vi "Tool detail GUI and STAT 2 collector.vi"(1 "Detail W1":u16, 2 "Detail W2":u16, 3 "LEIN contoller STAT2 data dekoder":i32, 11 "error in (no error)":errorcluster) -> ()   [LabVIEW 2011]
uses:
  Analog value.ctl
  Analog Var Disp 0 sif.ctl
  Status indicator Black Small.ctl
  Digital value.ctl
  Measurments Handling/Digital GUI/Digital Display cluster.ctl
  Measurments Handling/Digital GUI/Digital Disp small indicator.ctl
  Status indicator white.ctl
  Controls/Tristate/Tristate Valve state.ctl
  LEINmaster/Defenitions/LEIN STAT 15 Id system cluster v2.ctl
  LEINmaster/Defenitions/LEIN STAT 14 Debug system cluster.ctl
  LEINmaster/Defenitions/Error_system_def.ctl
  LEINmaster/Defenitions/LEIN stat 1 Stat defenition.ctl
  Tool/List of nodes in tool.ctl
  Tool/Stroker/STroker Raw value indicator.ctl
  LEINmaster/Nodes/Controller local stat2.ctl
  LEINmaster/Nodes/pressure stat2.ctl
  LEINmaster/Nodes/solonoid stat2.ctl
  LEINmaster/Nodes/PSU stat2.ctl
  LEINmaster/Nodes/tensionsub stat2.ctl
  LEINmaster/Status any node.ctl
  LEINmaster/Defenitions/stat2/system status/Stat2 system error.ctl
  LEINmaster/Defenitions/stat2/system status/Stat2 system task info.ctl
  Tool/Tab with tool type tabs.ctl
  LEINmaster/Defenitions/LEIN STAT 15 Id system cluster v2 wo lables.ctl
  <vilib>/Utility/miscctls.llb/LVStringsAndValuesArrayTypeDef.ctl
  emi cndiates/E&S/reate/S&E Event source.ctl
  Events/User Event List.ctl
  LEINmaster/Defenitions/LEIN Structure variations.ctl
  Solenoid Status Override.ctl
  LEINmaster/Defenitions/LEIN stat 14 module array.ctl
  Tool/Variable List Tool Digital.ctl
  Measurments Handling/Common/Variable List Common Analog.ctl
  Measurments Handling/Common/Variable List Common Digital.ctl
  Measurments Handling/Action Analog Handler.ctl
  emi Lib/System 01/0 - General/App/Loop control 2/Private/_emi_SMLoop Control Single.vi
  emi Lib/System 01/0 - General/emi_Read System ID.vi
  emi Lib/System 01/0 - General/App/Loop control 2/Private/_emi_ SMLoop start condition.vi
  emi Lib/System 01/0 - General/App/Loop control 2/Private/_emi_ SMLoop Error Check.vi
  emi Lib/System 01/0 - General/App/Loop control 2/Private/_emi_SMLoop Register new.vi
  emi Lib/System 01/0 - General/S&E reporting/emi_Send S&E Error message.vi
  emi Lib/Basic/0 - General/Error/emi_ Is Error state.vi
  emi Lib/System 01/0 - General/App/Loop control/Private/_emi_GFV Loop Running.vi
  emi Lib/System 01/0 - General/App/Loop control 2/Private/_emi_ SMLoop Restart Counter.vi
  emi Lib/System 01/0 - General/App/Loop control/Private/_emi_GFV stop a loop so it can reset.vi
  emi Lib/System 01/0 - General/App/Loop control 2/Private/_emi_ SMLoop Restart.vi
  emi Lib/System 01/0 - General/App/Loop control/Private/_emi_GFV Loop Linking.vi
  emi Lib/System 01/0 - General/App/Loop control/Private/_emi_GFV Loop Enable.vi
  emi Lib/System 01/0 - General/App/Private/_emi_GFV App Close.vi
  emi Lib/System 01/0 - General/Private/_emi_GFV System ID.vi
  emi Lib/System 01/0 - General/S&E reporting/Private/_emi_S&E Q Generator.vi
  <vilib>/Utility/VariantDataType/GetNumericInfo.vi
panel:
  in  "Close":bool
  out "Tool type:":string
  in  "Tab Control":T1(tab)
  out "Type tab 2":T2
  in  "Send stroker current pos new":bool caption="Solonoid 3 off"
  in  "Stroke pos (mm)":dbl format="%.1f"
  out "Anchor":T3 caption="Solonoid State Anchor"
  out "Solenoid State Stroker":T3 caption="Stroker direction"
  out "Solenoid State Master":T3 caption="Stroker enable"
  in  "Solonoid 1 On":bool
  in  "Solenoid 2 On":bool
  in  "Solenoid 3 On":bool
  in  "Solenoid 1 Off":bool
  in  "Solenoid 2 Off":bool
  in  "Solonoid 3 off":bool
  in  "Send stroker current pos":bool caption="Solonoid 3 off"
  in  "Stroke position to use(mm)":dbl format="%.1f"
  in  "Force ID update":bool caption="Solonoid 3 off"
  out "Main controller":T4 {"LEIN impl. code" format="%02x"; "Serial number" format="%04.0f"; "HW ID" format="%02x"; "FW ID" format="%02x"; "HW REV" format="%02x"; "FW REV" format="%02x"}
  out "Sub nodes":T5[](array[typedef]) {"LEIN implementation code" format="%.0x"; "Serial number" format="%04.0f"; "HW REV" format="%02x"}
  out "Node status array":T6[](array[typedef])
  out "Tool Raw values":T9 {"PSU"."sys register" format="%04x"; "Tension Sub 2"."sys register" format="%04x"; "Tension Sub 1"."sys register" format="%04x"; "Solenoid"."valve status" format="%02x"; "Solenoid"."sys register" format="%04x"; "pressure 2"."sys register" format="%04x"; "pressure 1"."sys register" format="%04x"; "Controller"."High G monitoring" format="%02x"; "Controller"."NA" format="%02x"; "Controller"."GPIO values" format="%02x"; "Controller"."Relay status" format="%02x"; "Controller"."sys register" format="%04x"}
  in  "Clear error":bool
  in  "Node":T15 items=["Stroker Main Controller", "Pressure node 1", "Pressure node 2", "Solenoid node", "PSU", "Tension Sub1", "Tension Sub2"]
  out "Debug received":bool
  out "Error received":bool
  out "Task received":bool
  out "Common Task status":T16
  out "Common error":T17 {"Module error mask" format="%08b"}
  in  "Get Task registers":bool
  in  "Get Error registers":bool
  in  "Get Debug registers":bool
  out "Common Debug data":T18
  out "Additional Task status":string
  out "Additional Error status":string
  out "Additional Debug status":string
  out "System digital values":T19[](array[typedef])
  out "System analog values":T23[](array[typedef]) {"val"."Value" format="%#.1f"}
  # "Direct solenoid control"
  # "Solenoid status override"
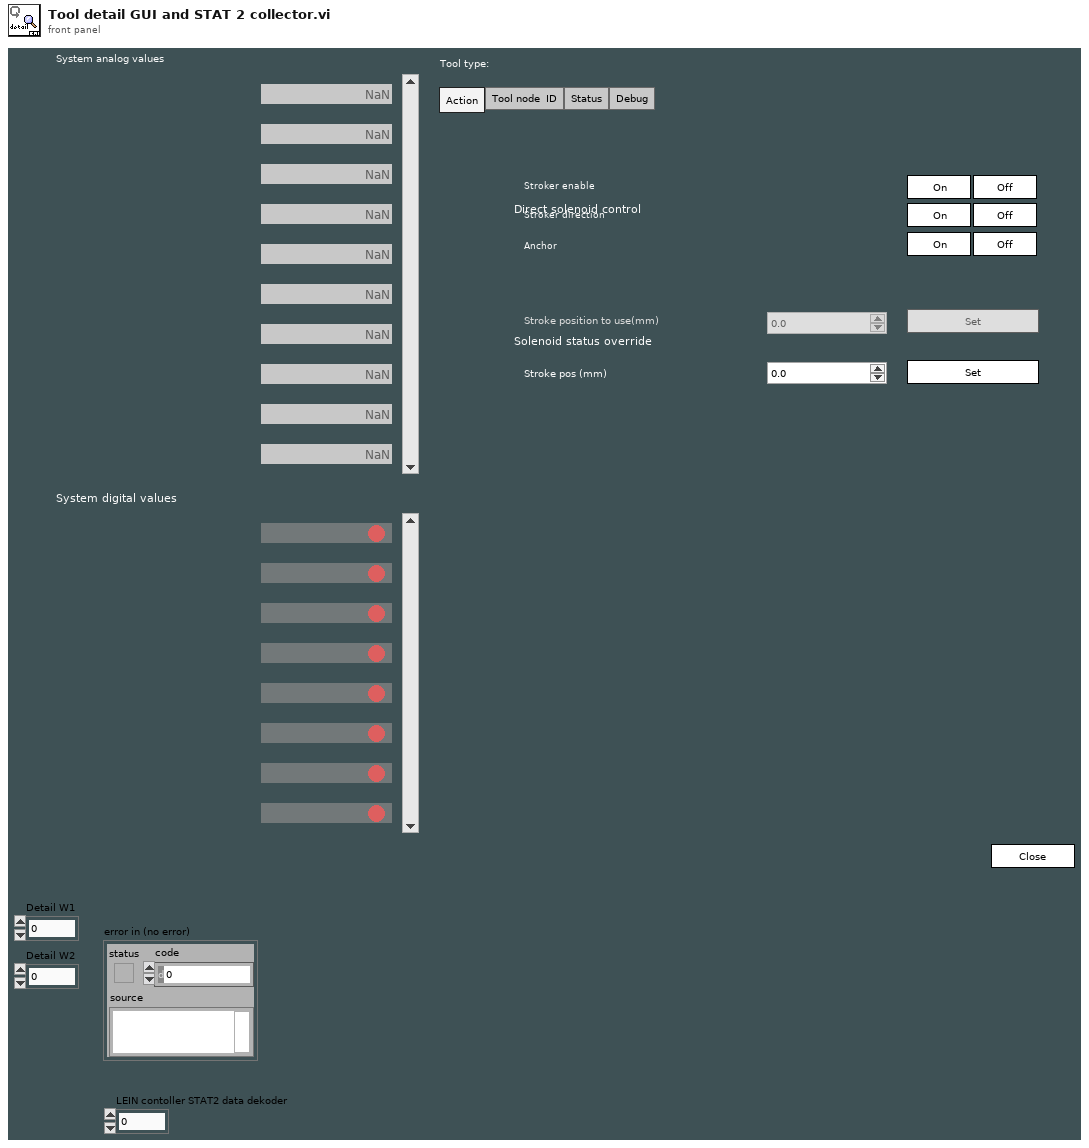
[diagram p1: front panel]
types:
  T1 = enum32{"Action", "Tool node  ID", "Status", "Debug"}
  T2 = typedef "Tab with tool type tabs.ctl" = enum32{"Stroker", "Driller", "Tractor"}
  T3 = typedef "Tristate Valve state.ctl" = u16
  T4 = typedef "LEIN STAT 15 Id system cluster v2.ctl" = cluster{"LEIN version":u8, "LEIN impl. code":u8, "Serial number":u16, "Project":u16, "HW ID":u8, "FW ID":u8, "HW REV":u8, "FW REV":u8}
  T5 = typedef "LEIN STAT 15 Id system cluster v2 wo lables.ctl" = cluster{"LEIN version":u8, "LEIN implementation code":u8, "Serial number":u16, "Project":u16, "HW ID":u8, "FW ID":u8, "HW REV":u8, "FW REV":u8}
  T6 = typedef "Status any node.ctl" = cluster{"Name":string, "Connected":bool, "Stopped":bool, "Error":T7, "Task":T8}
  T7 = typedef "Stat2 system error.ctl" = cluster{"Error":bool, "Has had error":bool, "Com. issue":bool}
  T8 = typedef "Stat2 system task info.ctl" = cluster{"Task":bool, "Task error":bool, "Task cnt.":u8, "Job 0":bool, "User":bool}
  T9 = typedef "STroker Raw value indicator.ctl" = cluster{"Controller":T10, "pressure 1":T11, "pressure 2":T11, "Solenoid":T12, "PSU":T13, "Tension Sub 1":T14, "Tension Sub 2":T14, "Pos override used":bool}
  T10 = typedef "Controller local stat2.ctl" = cluster{"sys register":u16, "temperature":u16, "Input voltage":u16, "Input Current":u16, "Accelerometer ch0":u16, "Accelerometer ch1":u16, "Accelerometer ch2":u16, "Relay status":u8, "GPIO values":u8, "Sensor 1":i32, "Sensor 2":i32, "NA":u8, "High G monitoring":u8}
  T11 = typedef "pressure stat2.ctl" = cluster{"sys register":u16, "temperature":u16, "Pressure":u16, "osctun":u8}
  T12 = typedef "solonoid stat2.ctl" = cluster{"sys register":u16, "temperature":u16, "Position":i16, "monitor state":u8, "valve status":u8}
  T13 = typedef "PSU stat2.ctl" = cluster{"sys register":u16, "temperature":u16, "HV Voltage in":u16, "Main Voltage out":u16, "Main Current out":u16}
  T14 = typedef "tensionsub stat2.ctl" = cluster{"sys register":u16, "temperature":u16, "Tension":i16, "osctun":u8}
  T15 = typedef "List of nodes in tool.ctl" = u16
  T16 = typedef "LEIN stat 1 Stat defenition.ctl" = cluster{"Task ID":u8, "Task counter":u8, "Task result code":u8, "reserved":u8}
  T17 = typedef "Error_system_def.ctl" = cluster{"Uptime(minutes)":u16, "Com state 1 (crc/Tx)":u8, "Com state 2 (bit timing /Rx)":u8, "System error code":u8, "Module error mask":u8}
  T18 = typedef "LEIN STAT 14 Debug system cluster.ctl" = cluster{"Max handler call interval":u16, "Messages received":u16, "Valid messages received":u16, "Replies sent":u16, "Nack sent":u16}
  T19 = typedef "Digital value.ctl" = cluster{"Name":string, "Val":T20}
  T20 = typedef "Digital Display cluster.ctl" = cluster{"ON/OFF TEXT":string, "Val":T21, "Status":T22}
  T21 = typedef "Digital Disp small indicator.ctl" = u16
  T22 = typedef "Status indicator white.ctl" = u16
  T23 = typedef "Analog value.ctl" = cluster{"Name":string, "val":T24}
  T24 = typedef "Analog Var Disp 0 sif.ctl" = cluster{"Value":dbl, "Unit":string, "Status":T25}
  T25 = typedef "Status indicator Black Small.ctl" = u16
  T26 = typedef "LVStringsAndValuesArrayTypeDef.ctl" = cluster{"String":string, "Value":ext}[]
  T27 = typedef "Variable List Tool Digital.ctl" = enum16{"Tool Error Controller", "Tool Stopped Controller", "Tool Relay 1", "Tool Relay 2", "Tool Both Relays", "Tool node Pressure 1", "Tool Error Pressure 1", "Tool Stopped Pressure 1", "Tool node Pressure 2", "Tool Error Pressure 2", "Tool Stopped Pressure 2", "Tool node Solenoid", "Tool Error Solenoid", "Tool Stopped Solenoid", "Tool Solenoid 1", "Tool Solenoid 2", "Tool Solenoid 3", "Tool node PSU", "Tool Error PSU", "Tool Stopped PSU", "Upper Tension Sub", "Tool Error Upper Tension Sub", "Tool Stopped Upper Tension Sub", "Lower Tension Sub", "Tool Error Lower Tension Sub", "Tool Stopped Lower Tension Sub", "Stroke Target seeking", "Stroke Moving Out", "Stroke Moving Inn", "Stroke valves set for Out", "Stroke valves set for In", "Stroke In (force)", "Stroke Out (force)", "Stroke Force decreasing(in)", "Stroke Force decreasing(out)", "Stroke Force change not correct", "Stroke SLIPS established P1", "Stroke SLIPS established P2", "Stroke SLIPS established", "Stroke Pressure Monitor Ongoing", "Stroke Pressure Monitor Ending ", "Tool Stroke enable Valve", "Tool Stroke direction Valve", "Tool Anchor Valve", "Stroker Var19 - Reserved", "Stroker Var20 - Reserved", "Stroker Var21 - Reserved", "Stroker Var22 - Reserved", "Stroker Var23 - Reserved", "Stroker Var24 - Reserved", "Tractor Var1 - Reserved", "Tractor Var2 - Reserved", "Tractor Var3 - Reserved", "Tractor Var4 - Reserved", "Tractor Var5 - Reserved", "Tractor Var6 - Reserved", "Tractor Var7 - Reserved", "Tractor Var8 - Reserved", "Oil filling mode", "Mill Bit Direction", "Position control", "Anchor", "Driller Var5 - Reserved", "Driller Var6 - Reserved", "Driller Var7 - Reserved", "Driller Var8 - Reserved"}
  T28 = typedef "S&E Event source.ctl" = enum16{"User", "Instrument", "Application", "Windows"}
  T29 = enum16{"big-endian, network order", "native, host order", "little-endian"}
  T30 = typedef "LEIN custom reply Q.ctl" = refnum<queue>
  T31 = typedef "_emi_ SMLoop sates.ctl" = enum16{"Init", "Standby", "Start", "Normal Operation", "Stop", "Error Handling", "End", "Post"}
  T32 = typedef "Options  All pages and custom.ctl" = cluster{"P 1 (App)":T33, "P 2":T34, "P 3":T35, "P 4":T38, "P 5":T43, "P 6 (Err)":T44, "P 7 (Expert)":T45, "P 8 (Depth)":T47, "C 1":T48, "C 2":T49}
  T33 = typedef "Options Page 1 (App).ctl" = cluster{"Result files":path, "PCP Interface":string, "Tractor/Stroker Interface":string, "Tractor Interface":string, "Modem Status Interface":string, "Audible Alarm":bool, "Force alarm on Technical":bool, "Force alarm on HH":bool, "Force alarm on LL":bool, "Force alarm on H":bool, "Force alarm on L":bool}
  T34 = typedef "Options Page 2.ctl" = cluster{"Solenoid & Relay latching time":u16, "Tractor relay 1":dbl, "Tractor relay 2":dbl, "Tractor Solenoid limit":dbl}
  T35 = typedef "Options Page 3.ctl" = cluster{"Min resistance":dbl, "Max resistance":dbl, "Head voltage range":T36, "Max voltage jump":dbl, "Maximum resistance change":dbl, "Start Telemetry Voltage":dbl, "Start Telemetry Timeout":dbl, "Start Motor Voltage":dbl, "Stop Motor Voltage":dbl, "Pass Mode Warning Voltage":dbl, "Relay Switch Voltage":dbl, "Relay Status Loss Voltage":dbl, "Samples to average":i32, "PSU type DO NOT USE":T37, "Magna OVP":dbl, "Magna Current Limit":dbl}
  T36 = typedef "PCP type List.ctl" = enum16{"0 - 350V", "0 - 450V", "0 - 600V"}
  T37 = typedef "PSU Type.ctl" = enum16{"Unipower", "Magna 8.3A", "Magna 12A", "None"}
  T38 = typedef "Options Page 4.ctl" = cluster{"Solenoid & Relay latching time":u16, "Stroker relay 1":dbl, "Stroker Relay 2":dbl, "Stroker Solenoid limit":dbl, "Force det.":T39, "Stroke force lim.":dbl, "Anchor Enabled Pressure":dbl, "Tacometer puls":dbl, "Default anchor behavior":T40, "Default stroker behavior":T41, "Default stroker force limit (tonne)":dbl, "Slips Size":T42}
  T39 = typedef "Stroke force selector.ctl" = enum16{"Stroke in = node 1", "Strok out = node 1"}
  T40 = typedef "Default anchor behavior.ctl" = enum16{"Do nothing", "Set Anchor", "Release Anchor"}
  T41 = typedef "Default stroker behavior.ctl" = enum16{"Do nothing", "Stop", "Go Out", "Go In"}
  T42 = typedef "Slips Type Radio.ctl" = enum32{"No Selection", "338 MRS", "3,9 MRS"}
  T43 = typedef "Options Page 5.ctl" = cluster{"Solenoid & Relay latching time":u16, "Driller relay 1":dbl, "Driller Relay 2":dbl, "Driller  Solenoid limit":dbl}
  T44 = typedef "Options Page 6 (Err).ctl" = cluster{"Error and event files":path}
  T45 = typedef "Options Page 7 (Expert).ctl" = cluster{"Show Debug":bool, "Log debug messages":bool, "Additional debug messages":bool, "Start Beagle with Simulator data":bool, "Workshop mode":bool, "Modem baud":u16, "enumCANCOM":bool, "Modem sim":T46, "Telemetry Timeout Disable":i32, "Buffer size":i32, "Upd regular data":bool, "Cable comp":cluster{"VMOD1 Voltage(V)":dbl, "VMOD2 Voltage(V)":dbl}}
  T46 = typedef "Modem simulation setup.ctl" = cluster{"Modem dealay sim":bool, "Sim baud Tx":u16, "Bit Error fraction Tx":dbl, "Sim baud Rx":u16, "Bit Error fraction Rx":dbl}
  T47 = typedef "Options Page 8 (Depth).ctl" = cluster{"Winch Spool Circumference":dbl, "Winch Pulses per Revolution":dbl, "Current Depth":dbl}
  T48 = typedef "Options Custom 1.ctl" = cluster{"Depth Updated":bool, "Depth Offset":dbl}
  T49 = typedef "Options Custom 2.ctl" = cluster{"Placeholder":bool}
  T50 = typedef "List of tools.ctl" = enum16{"Stroker", "Driller", "Tractor"}
  T51 = typedef "User Event List.ctl" = enum16{"ESCAPE", "HV ON", "HV OFF", "HV SP Start adjusting", "HV SP Adjusted", "Sequence Started", "Stop Tool Operation", "Start Telemetry Operation", "Start Motor Operation", "Stroker Activated", "Driller Activated", "Tractor Activated", "Reset Telemetry", "Stop Telemetry", "Stop Motor Operation", "Cable Resistance Updated", "Cable Resistance Update Failed", "String Check Recording Started", "String Check Recording Stopped", "STROKER tool: Stroke enable Solenoid ON", "STROKER tool: Stroke enable Solenoid OFF", "STROKER tool: Stroke direction Solenoid ON", "STROKER tool: Stroke direction Solenoid OFF", "STROKER tool: Anchor Solenoid ON", "STROKER tool: Anchor Solenoid OFF", "Stroker - Set force and pressure to ZERO", "Stroker - Set tension subs to ZERO", "Mono Relay ON - PASS mode", "Hepta Relay ON - PASS mode", "Mono Relay OFF - MOTOR mode", "Hepta Relay OFF - MOTOR mode", "Relays set to passenger mode", "Relays set to motor mode", "Tractor - Set Tension Subs to ZERO", "High-G monitoring Stop", "High-G data retreival requested", "High-G data stop retreival requested", "High-G data retreived", "STROKER tool: Stroker position override sent", "Stroker Stop", "Stroker Extend", "Stroker Retract", "Stroker go to Position", "Controller Stop command", "Node clear error", "STROKER tool: Stroke stop homing", "STROKER tool: Start Monitoring", "STROKER tool: Stop Monitoring", "Sequence start", "Sequence stop", "Sequence stopped", "Sequence step approved", "Sequence action", "Failed sequence step, Retry", "Failed sequence step, Continue", "Failed sequence step, Abort", "Run Started", "Run Stopped"}
  T52 = typedef "LEIN Structure variations.ctl" = enum16{"LEIN08", "LEIN31", "LEIN63"}
  T53 = typedef "LEIN CMD Cluster.ctl" = cluster{"SID":u8, "ANF":bool, "CMD":T54, "DATA":u8[]}
  T54 = typedef "LEIN CMD List.ctl" = enum8{"ACTI", "TASK", "RES0", "STAT", "RES1", "RES2", "RES3", "USER"}
  T55 = typedef "Solenoid Status Override.ctl" = u8
  T56 = typedef "LEIN stat 14 module array.ctl" = u8[]
  T57 = typedef "Expected STAT lenght cluster.ctl" = cluster{"LEIN 0(error)":u16, "LEIN 1(Task)":u16, "LEIN 2(stat2)":u16, "LEIN 14(Debug)":u16, "LEIN 15(ID)":u16}
  T58 = typedef "Status Digitalish.ctl" = enum16{"NA", "False", "True"}
  T59 = typedef "Fixed Analog Channel Definition.ctl" = cluster{"ID":u16, "Name":string, "Quantity":T60, "Unit":string, "Maximum upd":T61, "Comment":string, "Help file Name":string, "Help file Section ":string, "Category":T62, "User adjustable Scaling":bool, "Default Scaling":T63, "Default Unit":i32, "Classification":T64}
  T60 = typedef "Quantity enum.ctl" = enum16{"NA", "Acceleration", "Angle", "Current", "Force", "Distance", "Pressure", "Resistance", "Rotational Speed", "Speed", "Temperature", "Tension", "Torque", "Voltage", "Weight"}
  T61 = typedef "Update frequensies.ctl" = enum16{"2 Hz", "1 Hz", "0.1 Hz"}
  T62 = typedef "Channel catagory Enum.ctl" = enum16{"No Category", "Power", "Temperature", "Pressure"}
  T63 = typedef "Scaling.ctl" = cluster{"Gain":dbl, "Offset":dbl}
  T64 = typedef "Channel Classification Enum.ctl" = enum16{"Basic", "Advanced", "Expert", "Unused"}
  T65 = typedef "Fixed Digital Channel Definition.ctl" = cluster{"ID":u16, "Name":string, "NA Text":string, "Off Text":string, "On Text":string, "Maximum upd":T61, "Comment":string, "Help file Name":string, "Help file Section ":string, "Catagory":T62, "In use":bool}
  T66 = typedef "Variable List Common Digital.ctl" = enum16{"PCP Connected", "PCP PC Control", "HV PSU connected", "HV PSU HV Active", "Modem Connected", "Tool Connected", "CanBus interface"}
  T67 = typedef "Variable List Common Analog.ctl" = enum16{"HVPSU Head Voltage", "HVPSU TS Voltage", "HVPSU Current", "PCP Cable Resistance", "Winch Depth", "Winch Line Speed", "Winch Wire Tension"}
  T68 = typedef "Action Analog Handler.ctl" = enum16{"GET value", "GET Single Frequenzy", "GET All Values", "GET Waveform", "Get Numb Var", "SET Value", "START Buffer", "REG Variable", "BUF size(total antal sekund)", "PULS", "Get a Value at time", "Set initial waveform"}
  T69 = cluster{"notifier out":refnum<notifier>, "Ana com":i32, "Dig com":i32, "Time of last valid tool data":u32}
  T70 = typedef "STAT2 data carrier type aware.ctl" = cluster{"Tool":T50, "Data":variant}
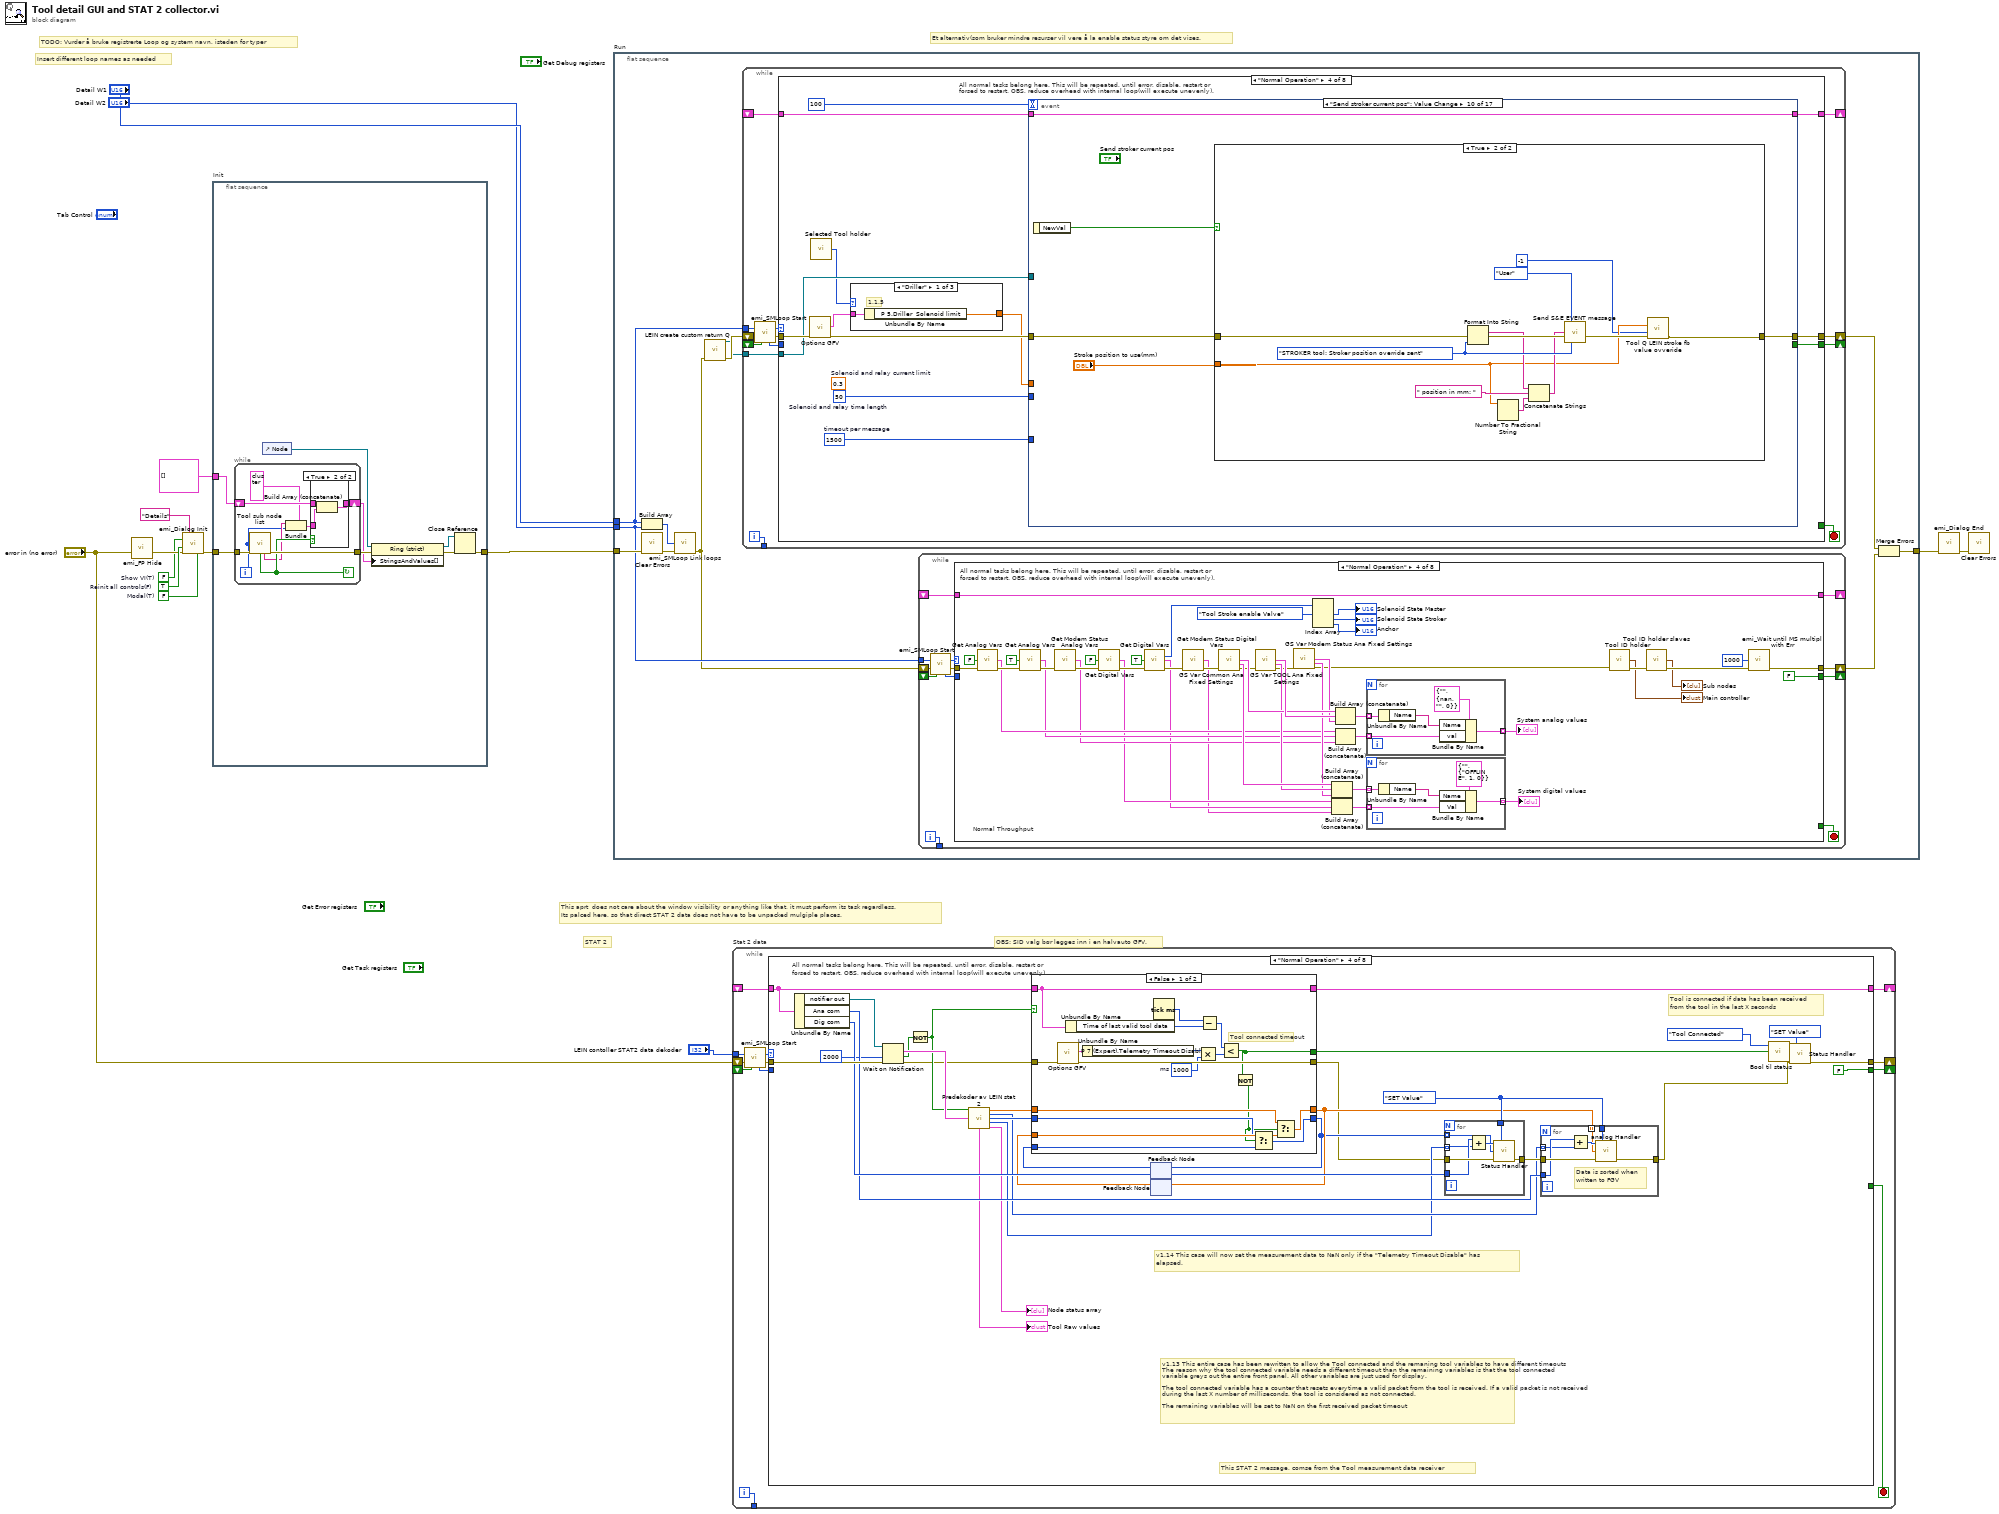
[diagram p0: block diagram]
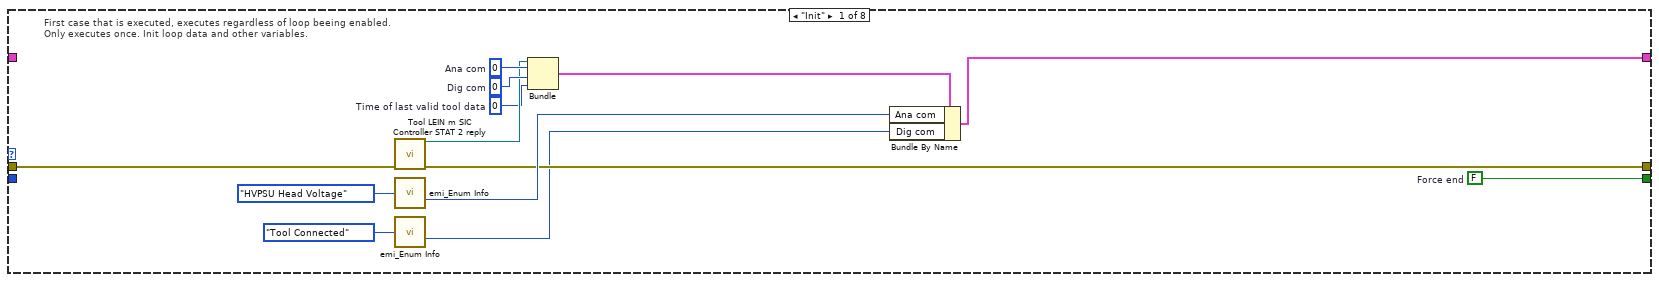
[diagram p2: hidden frame]
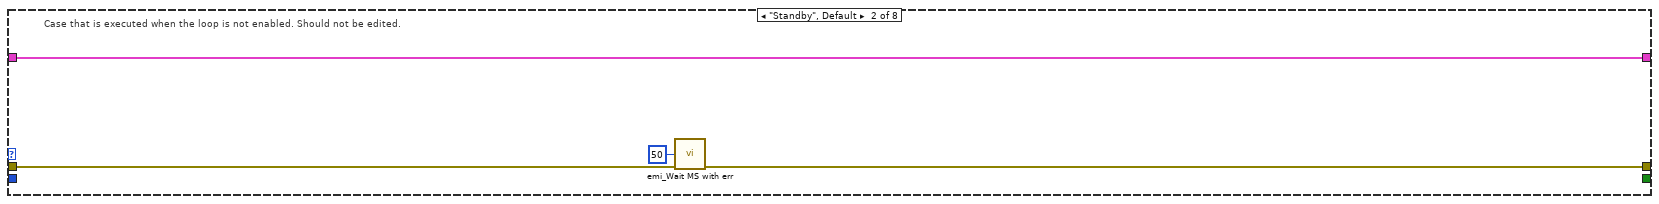
[diagram p3: hidden frame]
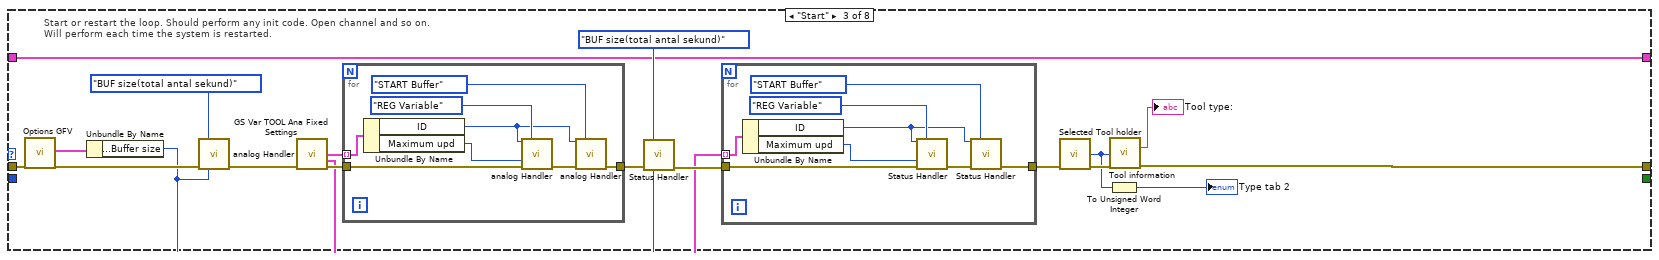
[diagram p4: hidden frame]
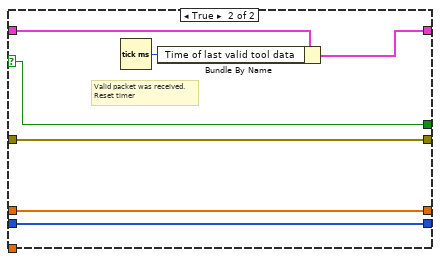
[diagram p5: hidden frame]
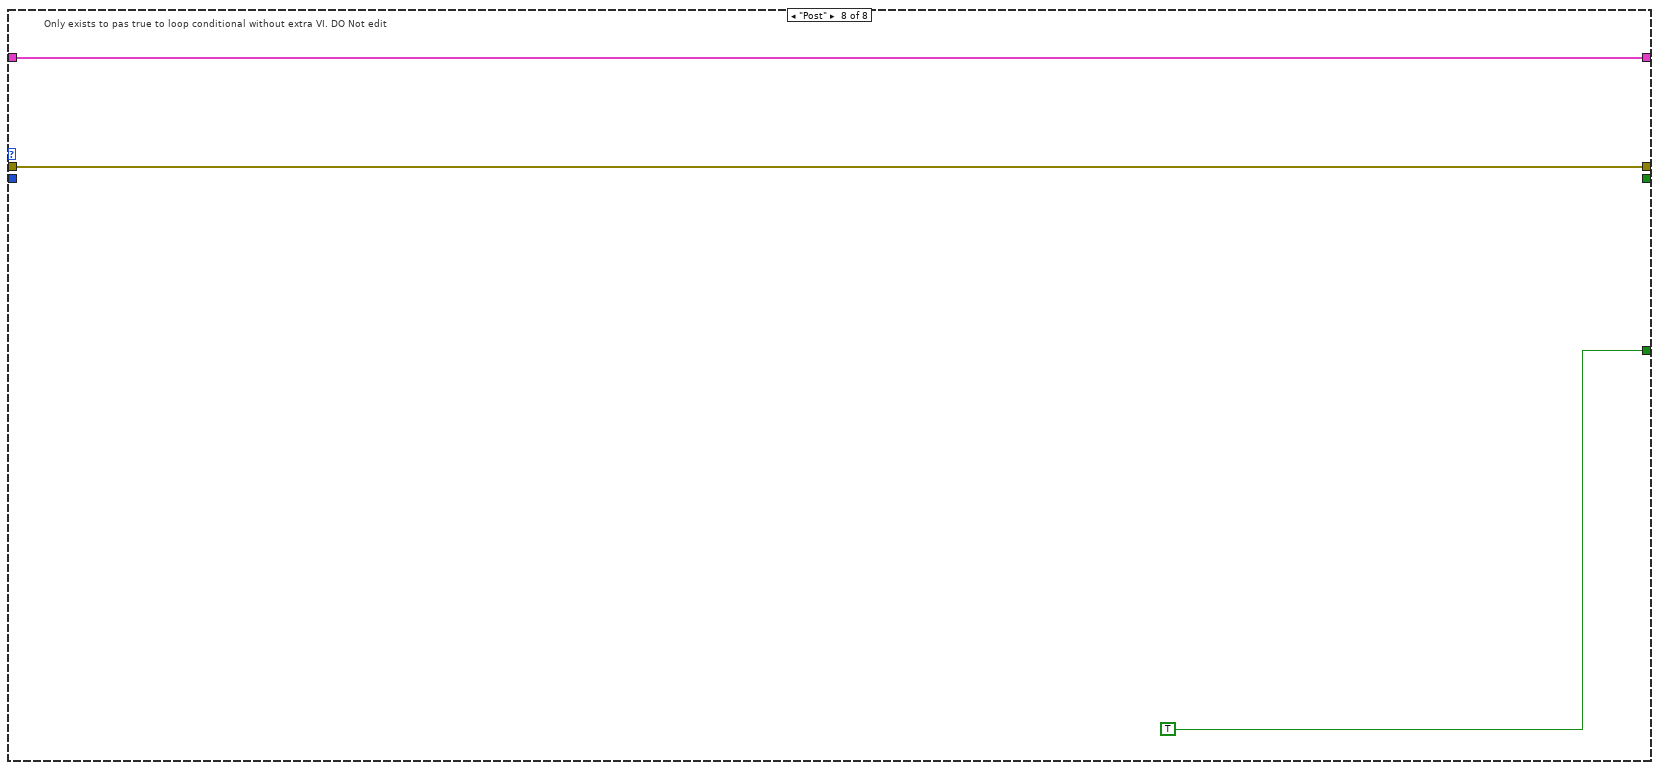
[diagram p9: hidden frame]
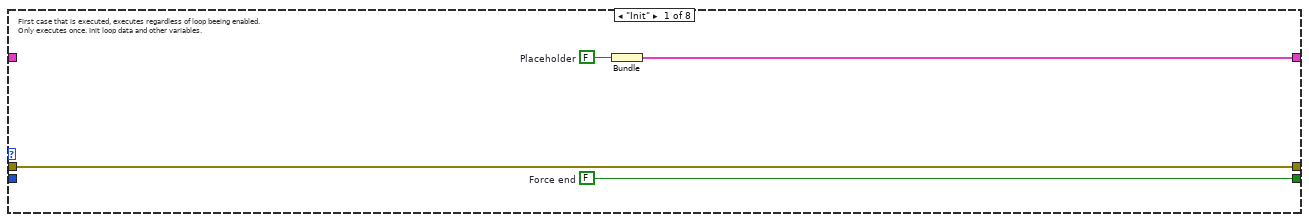
[diagram p11: hidden frame]
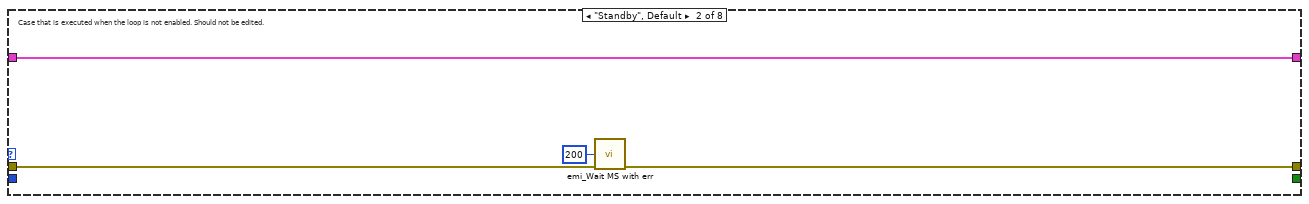
[diagram p12: hidden frame]
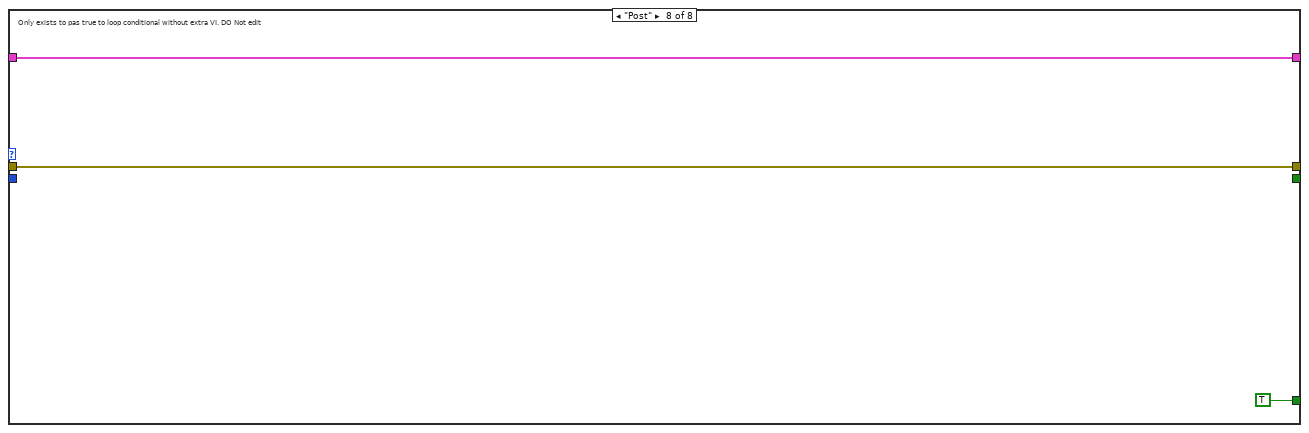
[diagram p17: hidden frame]
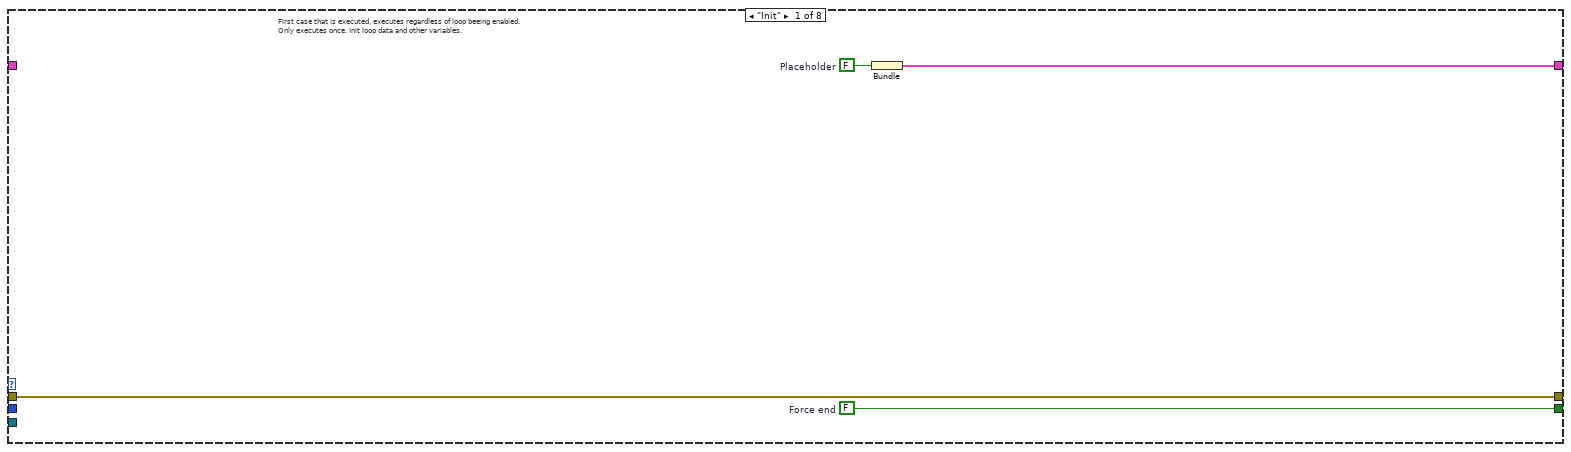
[diagram p18: hidden frame]
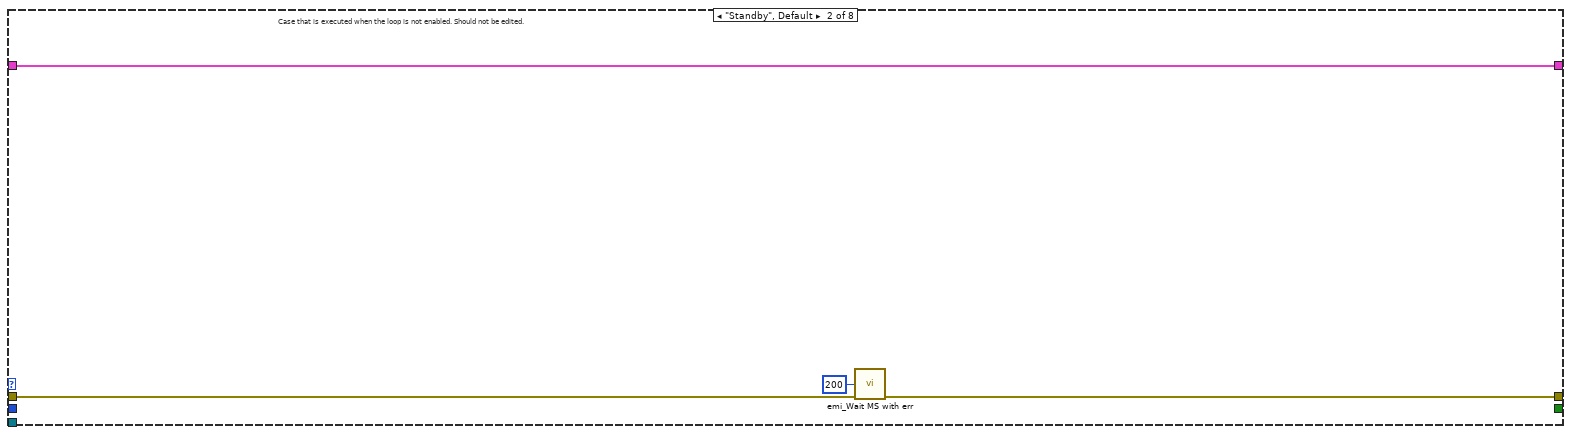
[diagram p19: hidden frame]
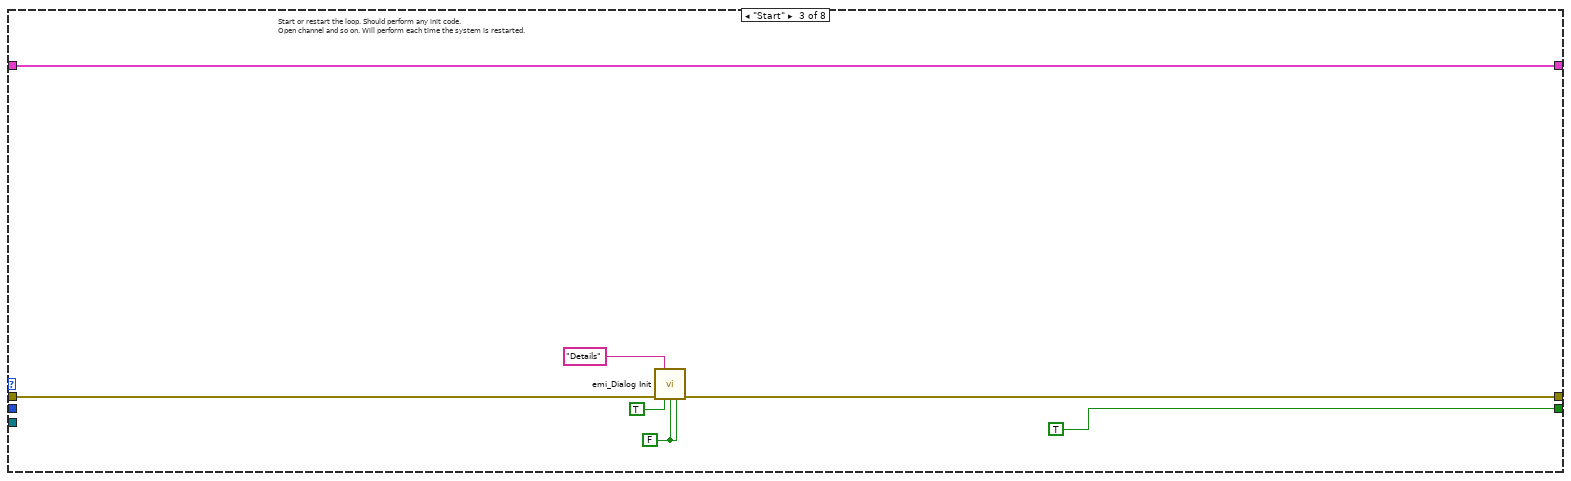
[diagram p20: hidden frame]
diagram:
  w9 = FALSE  # Show VI(T)
  w12 = TRUE  # Reinit all controls(F)
  w13 = FALSE  # Modal(T)
  # "This aprt  does not care about the window visibility or anything like that, it must perform its task regardless.\nIts palced here, so that direct STAT 2 data does not have to be unpacked mulgiple places."
  # "STAT 2"
  # "OBS: SID valg bør legges inn i en halvauto GFV."
  # "Et alternativ(som bruker mindre resurser vil vere å la enable status styre om det vises."
  # "TODO: Vurder å bruke registrerte Loop og system navn, isteden for typer"
  # "Insert different loop names as needed"
  n1 = call "emi_FP Hide.vi"("error in (no error)"="error in (no error)") -> ("error out"=w11:errorcluster)  [unwired: 13 in, 1 out]
  n2 = call "emi_Dialog Init.vi"("Header String(\"\")"="Details" ("Header String(\"\")"), "Show VI(T)"=w9, "Reinit all controls(F)"=w12, "error in"=w11, "Modal(T)"=w13) -> ("error out"=w10:errorcluster)  [unwired: 10 in]
  n3 = flat-sequence "Init" {
    tunnel: [w20] -> w7
    tunnel: w10 -> [w17]
    tunnel: T26 [] ("Strings And Values []") -> [w16]
    frame #0 {
      n4 = while {
        tunnel: [w30] -> w18
        tunnel: w17 -> [w31]
        shift-right: [w28] -> w15
        shift-left: w16 -> [w27]
        i -> [w24]
        stop <- w29 continue-if-true
        n5 = call "Tool sub node list.vi"("Tool node"=w24, "error in (no error)"=w31) -> ("node registered"=w29:bool, "Node name"=w25:string, "error out"=w30:errorcluster)  [unwired: 6 in, 5 out]
        n6 = Bundle(cluster=cluster{"String":string, "Value":ext} {"String"="", "Value"=0.0}, "String"=w25, "Value"=w24) -> (w23:cluster{"String":string, "Value":ext})
        n7 = case shown="True" w29 {
          tunnel: [w32 w34] -> w28
          tunnel: w27 -> [w32 w35]
          tunnel: w23 -> [_ w33]
          frame False {
          }
          frame True {
            n8 = Build Array (concatenate)(w35, w33) -> (w34:T26)
          }
        }
      }
      n9 = control-ref of="Node"() -> (w19:refnum<vi>)
      n10 = property class="Ring (strict)"(reference=w19, error in=w18, "StringsAndValues[]"=w15) -> (reference out=w21:refnum<vi>, error out=w22:errorcluster)
      n11 = Close Reference(reference=w21, error in (no error)=w22) -> (error out=w20:errorcluster)
    }
  }
  n12 = flat-sequence "Run" {
    tunnel: w7 -> [w46]
    tunnel: [w43] -> w8
    tunnel: "Detail W1" -> [w41]
    tunnel: "Detail W2" -> [w40]
    frame #0 {
      n13 = Build Array(w41, w40) -> (w39:u16[])
      n14 = call <vilib>:"Clear Errors.vi"("error in (no error)"=w46) -> ("error out"=w42:errorcluster)  [unwired: 6 in]
      n15 = call "emi_SMLoop Link loops.vi"("Loop IDS"=w39, "error in (no error)"=w42) -> ("error out"=w38:errorcluster)  [unwired: 13 in]
      n16 = call "LEIN create custom return Q.vi"("error in (no error)"=w38) -> ("LEIN custom reply Q"=w36:T30, "error out"=w37:errorcluster)  [unwired: 13 in]
      n17 = while {
        shift-right: [w145] -> _
        shift-left: _ -> [w141]
        shift-right: [w143] -> w45
        shift-left: w37 -> [w139]
        tunnel: [w142] -> _
        shift-right: [w140] -> _
        shift-left: _ -> [w135]
        tunnel: w41 -> [w136]
        tunnel: w36 -> [w133]
        i -> [w142]
        stop <- w144 stop-if-true
        n18 = call "emi_SMLoop Start.vi"("Loop ID"=w136, "error in (no error)"=w139, "Force Stop(F)"=w135) -> ("Loop command"=w137:T31, "error out"=w138:errorcluster, "Loop ID out"=w134:i32)  [unwired: 10 in]
        n19 = case shown="\"Normal Operation\"" w137 {
          tunnel: [w148 w150 w160 w171 w565 w580 w581 w584] -> w145
          tunnel: [_ _ _ _ _ _ _ TRUE] -> w144
          tunnel: w138 -> [w149 w152 w158 w173 w564 w579 w582 w585]
          tunnel: [w149 w151 w159 w172 w560 w579 w582 w585] -> w143
          tunnel: w141 -> [_ w150 w160 w170 w565 w580 w581 w584]
          tunnel: [w146 _ TRUE ("Discard?") w169 _ _ _ _] -> w140
          tunnel: w134 -> [_ _ _ _ w563 _ _ _]
          tunnel: w133 -> [_ _ _ w168 _ _ _ _]
          frame "Init" {
            w146 = FALSE  # Force end
            w147 = FALSE  # Placeholder
            # "First case that is executed, executes regardless of loop beeing enabled.\nOnly executes once. Init loop data and other variables."
            n20 = Bundle("Placeholder"=w147) -> (w148:cluster{"Placeholder":bool})  [unwired: 1 in]
          }
          frame "Standby", Default {
            # "Case that is executed when the loop is not enabled. Should not be edited."
            n21 = call "emi_Wait MS with err.vi"("milliseconds to wait(0)"=u32 200, "error in (no error)"=w152) -> ("error out"=w151:errorcluster)  [unwired: 13 in]
          }
          frame "Start" {
            w155 = FALSE ("Set BG Color(T)")
            # "Start or restart the loop. Should perform any init code. \nOpen channel and so on. Will perform each time the system is restarted."
            n22 = call "emi_Dialog Init.vi"("Header String(\"\")"="Details" ("Header String(\"\")"), "error in"=w158, "Center in bottom FP(T)"=TRUE, "Set BG Color(T)"=w155, "Modal(T)"=w155) -> ("error out"=w159:errorcluster)  [unwired: 10 in]
          }
          frame "Normal Operation" {
            w165 = 1500  # timeout per message
            w166 = u16 50  # Solenoid and relay time length
            (unwired) 0.3  # Solenoid and relay current limit
            # "All normal tasks belong here. This will be repeated, until error, disable, restart or\nforsed to restart. OBS, reduce overhead with internal loop(will execute unevenly)."
            n23 = call "Options GFV.vi"("error in (no error)"=w173) -> ("Options"=w163:T32, "error out"=w164:errorcluster)  [unwired: 16 in, 1 out]
            n24 = call "Selected Tool holder.vi"() -> ("Tool out"=w161:T50)  [unwired: 14 in, 1 out]
            n25 = case shown="\"Driller\"" w161 {
              tunnel: w163 -> [w175 w177 w179]
              tunnel: [w174 w176 w178] -> w162
              frame "Driller" {
                # "1.1.5"
                n26 = Unbundle By Name(w175) -> ("P 5.Driller  Solenoid limit"=w174:dbl)
              }
              frame "Tractor" {
                # "1.1.5"
                n27 = Unbundle By Name(w177) -> ("P 2.Tractor relay 2"=w176:dbl)
              }
              frame "Stroker" {
                # "1.1.5"
                n28 = Unbundle By Name(w179) -> ("P 4.Stroker Solenoid limit"=w178:dbl)
              }
            }
            n29 = event shown="[9] \"Send stroker current pos\": Value Change" {
              selector: _ -> [_ _ _ _ _ _ _ _ _ _ _ _ _ _ _ _ _]
              dyn-events: _ -> [_ _ _ _ _ _ _ _ _ _ _ _ _ _ _ _ _]
              timeout: 100 -> [_ _ _ _ _ _ _ _ _ _ _ _ _ _ _ _ _]
              tunnel: w164 -> [w180 w184 w189 w211 w233 w255 w274 w299 w321 w350 w368 w395 w401 w448 w495 w515 w558]
              tunnel: w170 -> [w182 w185 w191 w213 w235 w257 w279 w301 w323 w352 w370 w396 w403 w450 w497 w517 w559]
              tunnel: [w182 w185 w191 w213 w235 w257 w279 w301 w323 w352 w370 w396 w403 w450 w497 w517 w559] -> w171
              tunnel: [w180 w184 w190 w212 w234 w256 w278 w300 w322 w351 w369 w395 w402 w449 w496 w516 w558] -> w172
              tunnel: [w181 w183 _ _ _ _ _ _ _ _ _ _ _ _ _ _ _] -> w169
              tunnel: w162 -> [_ _ w187 w209 w231 w253 w276 w297 w319 _ _ _ _ _ _ _ _]
              tunnel: w166 -> [_ _ w186 w208 w230 w252 w275 w296 w318 _ _ _ _ _ _ _ _]
              tunnel: w168 -> [_ _ _ _ _ _ _ _ _ _ _ _ w399 w446 w493 w513 _]
              tunnel: w165 -> [_ _ _ _ _ _ _ _ _ _ _ _ w398 w445 w492 w512 _]
              event Panel Close? {
                w181 = TRUE ("Discard?")
                # "Ellers varierer det om \nDebug Synlig/ikke Synlig huskes(\nalt etter om options vises etterpå)"
                n30 = event-data() -> ()  [unwired: 1 in, 3 out]
                n31 = event-data("Discard?"=w181) -> ()  [unwired: 1 in, 1 out]
              }
              event "Close": Value Change {
                n32 = event-data() -> ("NewVal"=w183:bool)  [unwired: 1 in]
              }
              event "Solenoid 1 Off": Value Change {
                n33 = event-data() -> ("NewVal"=w188:bool)  [unwired: 1 in]
                n34 = case shown="False" w188 {
                  tunnel: [w192 w206] -> w190
                  tunnel: w189 -> [w192 w199]
                  tunnel: w187 -> [_ w205]
                  tunnel: w186 -> [_ w204]
                  frame False {
                  }
                  frame True {
                    w197 = T15 3 items=["Main Controller", "Pressure node 1", "Pressure node 2", "Solenoid node"] ("Node")
                    w200 = User_Event_List."STROKER tool: Stroke enable Solenoid OFF" ("User Events")
                    n35 = Format Into String(error in=w199, w200) -> (resulting string=w201:string, error out=w202:errorcluster)  [unwired: 2 in]
                    n36 = call "Send S&E EVENT message.vi"("Event Source(user)"=S&E_Event_source."User", "Event Description"=w201, "error in (no error)"=w202, "Loc Sub ID/Event ID(No ID)"=w200) -> ("error out"=w198:errorcluster)  [unwired: 10 in, 1 out]
                    n37 = call "Selected Tool holder.vi"() -> ("Tool out"=w196:T50, "error out"=w195:errorcluster)  [unwired: 14 in]
                    n38 = call "Tool information.vi"("Tool in"=w196, "error in (no error)"=w195) -> ("Main node address"=w193:u8)  [unwired: 10 in, 3 out]
                    n39 = call "Tool sub node list.vi"("Tool node"=w197) -> ("SID"=w194:u8)  [unwired: 7 in, 7 out]
                    n40 = call "Tool Q LEIN solonoid valve task.vi"("Main Controller ID"=w193, "Solonoid ID"=w194, "current limit(0.2A)"=w205, "outpuyt channel"=u8 1, "time (50 ms)"=w204, "error in (no error)"=w198) -> ("error out"=w206:errorcluster)  [unwired: 8 in, 1 out]
                  }
                }
              }
              event "Solonoid 1 On": Value Change {
                n41 = event-data() -> ("NewVal"=w210:bool)  [unwired: 1 in]
                n42 = case shown="True" w210 {
                  tunnel: [w214 w228] -> w212
                  tunnel: w211 -> [w214 w221]
                  tunnel: w209 -> [_ w227]
                  tunnel: w208 -> [_ w226]
                  frame False {
                  }
                  frame True {
                    w219 = T15 3 items=["Main Controller", "Pressure node 1", "Pressure node 2", "Solenoid node"] ("Node")
                    w222 = User_Event_List."STROKER tool: Stroke enable Solenoid ON" ("User Events")
                    n43 = call "Selected Tool holder.vi"() -> ("Tool out"=w217:T50, "error out"=w216:errorcluster)  [unwired: 14 in]
                    n44 = call "Tool information.vi"("Tool in"=w217, "error in (no error)"=w216) -> ("Main node address"=w215:u8)  [unwired: 10 in, 3 out]
                    n45 = Format Into String(error in=w221, w222) -> (resulting string=w223:string, error out=w224:errorcluster)  [unwired: 2 in]
                    n46 = call "Send S&E EVENT message.vi"("Event Source(user)"=S&E_Event_source."User", "Event Description"=w223, "error in (no error)"=w224, "Loc Sub ID/Event ID(No ID)"=w222) -> ("error out"=w220:errorcluster)  [unwired: 10 in, 1 out]
                    n47 = call "Tool sub node list.vi"("Tool node"=w219) -> ("SID"=w218:u8)  [unwired: 7 in, 7 out]
                    n48 = call "Tool Q LEIN solonoid valve task.vi"("Main Controller ID"=w215, "Solonoid ID"=w218, "current limit(0.2A)"=w227, "outpuyt channel"=u8 0, "time (50 ms)"=w226, "error in (no error)"=w220) -> ("error out"=w228:errorcluster)  [unwired: 8 in, 1 out]
                  }
                }
              }
              event "Solenoid 2 On": Value Change {
                n49 = event-data() -> ("NewVal"=w232:bool)  [unwired: 1 in]
                n50 = case shown="True" w232 {
                  tunnel: [w236 w250] -> w234
                  tunnel: w233 -> [w236 w243]
                  tunnel: w231 -> [_ w249]
                  tunnel: w230 -> [_ w248]
                  frame False {
                  }
                  frame True {
                    w241 = T15 3 items=["Main Controller", "Pressure node 1", "Pressure node 2", "Solenoid node"] ("Node")
                    w244 = User_Event_List."STROKER tool: Stroke direction Solenoid ON" ("User Events")
                    n51 = call "Selected Tool holder.vi"() -> ("Tool out"=w240:T50, "error out"=w239:errorcluster)  [unwired: 14 in]
                    n52 = call "Tool sub node list.vi"("Tool node"=w241) -> ("SID"=w238:u8)  [unwired: 7 in, 7 out]
                    n53 = call "Tool information.vi"("Tool in"=w240, "error in (no error)"=w239) -> ("Main node address"=w237:u8)  [unwired: 10 in, 3 out]
                    n54 = Format Into String(error in=w243, w244) -> (resulting string=w245:string, error out=w246:errorcluster)  [unwired: 2 in]
                    n55 = call "Send S&E EVENT message.vi"("Event Source(user)"=S&E_Event_source."User", "Event Description"=w245, "error in (no error)"=w246, "Loc Sub ID/Event ID(No ID)"=w244) -> ("error out"=w242:errorcluster)  [unwired: 10 in, 1 out]
                    n56 = call "Tool Q LEIN solonoid valve task.vi"("Main Controller ID"=w237, "Solonoid ID"=w238, "current limit(0.2A)"=w249, "outpuyt channel"=u8 2, "time (50 ms)"=w248, "error in (no error)"=w242) -> ("error out"=w250:errorcluster)  [unwired: 8 in, 1 out]
                  }
                }
              }
              event "Solenoid 2 Off": Value Change {
                n57 = event-data() -> ("NewVal"=w254:bool)  [unwired: 1 in]
                n58 = case shown="True" w254 {
                  tunnel: [w258 w272] -> w256
                  tunnel: w255 -> [w258 w265]
                  tunnel: w253 -> [_ w271]
                  tunnel: w252 -> [_ w270]
                  frame False {
                  }
                  frame True {
                    w263 = T15 3 items=["Main Controller", "Pressure node 1", "Pressure node 2", "Solenoid node"] ("Node")
                    w266 = User_Event_List."STROKER tool: Stroke direction Solenoid OFF" ("User Events")
                    n59 = call "Selected Tool holder.vi"() -> ("Tool out"=w262:T50, "error out"=w261:errorcluster)  [unwired: 14 in]
                    n60 = call "Tool sub node list.vi"("Tool node"=w263) -> ("SID"=w260:u8)  [unwired: 7 in, 7 out]
                    n61 = call "Tool information.vi"("Tool in"=w262, "error in (no error)"=w261) -> ("Main node address"=w259:u8)  [unwired: 10 in, 3 out]
                    n62 = Format Into String(error in=w265, w266) -> (resulting string=w267:string, error out=w268:errorcluster)  [unwired: 2 in]
                    n63 = call "Send S&E EVENT message.vi"("Event Source(user)"=S&E_Event_source."User", "Event Description"=w267, "error in (no error)"=w268, "Loc Sub ID/Event ID(No ID)"=w266) -> ("error out"=w264:errorcluster)  [unwired: 10 in, 1 out]
                    n64 = call "Tool Q LEIN solonoid valve task.vi"("Main Controller ID"=w259, "Solonoid ID"=w260, "current limit(0.2A)"=w271, "outpuyt channel"=u8 3, "time (50 ms)"=w270, "error in (no error)"=w264) -> ("error out"=w272:errorcluster)  [unwired: 8 in, 1 out]
                  }
                }
              }
              event "Solenoid 3 On": Value Change {
                n65 = event-data() -> ("NewVal"=w277:bool)  [unwired: 1 in]
                n66 = case shown="True" w277 {
                  tunnel: [w280 w294] -> w278
                  tunnel: w274 -> [w280 w286]
                  tunnel: w276 -> [_ w293]
                  tunnel: w275 -> [_ w292]
                  frame False {
                  }
                  frame True {
                    w285 = T15 3 items=["Main Controller", "Pressure node 1", "Pressure node 2", "Solenoid node"] ("Node")
                    w288 = User_Event_List."STROKER tool: Anchor Solenoid ON" ("User Events")
                    n67 = call "Selected Tool holder.vi"() -> ("Tool out"=w284:T50, "error out"=w283:errorcluster)  [unwired: 14 in]
                    n68 = call "Tool sub node list.vi"("Tool node"=w285) -> ("SID"=w282:u8)  [unwired: 7 in, 7 out]
                    n69 = call "Tool information.vi"("Tool in"=w284, "error in (no error)"=w283) -> ("Main node address"=w281:u8)  [unwired: 10 in, 3 out]
                    n70 = Format Into String(error in=w286, w288) -> (resulting string=w289:string, error out=w290:errorcluster)  [unwired: 2 in]
                    n71 = call "Send S&E EVENT message.vi"("Event Source(user)"=S&E_Event_source."User", "Event Description"=w289, "error in (no error)"=w290, "Loc Sub ID/Event ID(No ID)"=w288) -> ("error out"=w287:errorcluster)  [unwired: 10 in, 1 out]
                    n72 = call "Tool Q LEIN solonoid valve task.vi"("Main Controller ID"=w281, "Solonoid ID"=w282, "current limit(0.2A)"=w293, "outpuyt channel"=u8 4, "time (50 ms)"=w292, "error in (no error)"=w287) -> ("error out"=w294:errorcluster)  [unwired: 8 in, 1 out]
                  }
                }
              }
              event "Solonoid 3 off": Value Change {
                n73 = event-data() -> ("NewVal"=w298:bool)  [unwired: 1 in]
                n74 = case shown="True" w298 {
                  tunnel: [w302 w316] -> w300
                  tunnel: w299 -> [w302 w309]
                  tunnel: w297 -> [_ w315]
                  tunnel: w296 -> [_ w314]
                  frame False {
                  }
                  frame True {
                    w307 = T15 3 items=["Main Controller", "Pressure node 1", "Pressure node 2", "Solenoid node"] ("Node")
                    w310 = User_Event_List."STROKER tool: Anchor Solenoid OFF" ("User Events")
                    n75 = call "Selected Tool holder.vi"() -> ("Tool out"=w306:T50, "error out"=w305:errorcluster)  [unwired: 14 in]
                    n76 = Format Into String(error in=w309, w310) -> (resulting string=w311:string, error out=w312:errorcluster)  [unwired: 2 in]
                    n77 = call "Tool information.vi"("Tool in"=w306, "error in (no error)"=w305) -> ("Main node address"=w303:u8)  [unwired: 10 in, 3 out]
                    n78 = call "Send S&E EVENT message.vi"("Event Source(user)"=S&E_Event_source."User", "Event Description"=w311, "error in (no error)"=w312, "Loc Sub ID/Event ID(No ID)"=w310) -> ("error out"=w308:errorcluster)  [unwired: 10 in, 1 out]
                    n79 = call "Tool sub node list.vi"("Tool node"=w307) -> ("SID"=w304:u8)  [unwired: 7 in, 7 out]
                    n80 = call "Tool Q LEIN solonoid valve task.vi"("Main Controller ID"=w303, "Solonoid ID"=w304, "current limit(0.2A)"=w315, "outpuyt channel"=u8 5, "time (50 ms)"=w314, "error in (no error)"=w308) -> ("error out"=w316:errorcluster)  [unwired: 8 in, 1 out]
                  }
                }
              }
              event "Force ID update": Value Change {
                n81 = event-data() -> ("NewVal"=w320:bool)  [unwired: 1 in]
                n82 = case shown="True" w320 {
                  tunnel: [w324 w332] -> w322
                  tunnel: w321 -> [w324 w331]
                  tunnel: w319 -> [_ _]
                  tunnel: w318 -> [_ _]
                  frame False {
                  }
                  frame True {
                    w338 = u16 60 ("Expected LEN")
                    w337 = LEIN_Structure_variations."LEIN63" ("LEIN Variation")
                    n83 = call "Get node version Q.vi"("error in"=w331) -> ("LEIN custom reply Q"=w330:T30, "error out"=w327:errorcluster)  [unwired: 13 in]
                    n84 = call "Selected Tool holder.vi"("error in (no error)"=w327) -> ("Tool out"=w329:T50, "error out"=w328:errorcluster)  [unwired: 13 in]
                    n85 = call "Tool information.vi"("Tool in"=w329, "error in (no error)"=w328) -> ("Main node address"=w325:u8, "error out"=w326:errorcluster)  [unwired: 10 in, 2 out]
                    n86 = call "LEIN CMD read STATs by len.vi"("SID"=w325, "LEIN Variation"=w337, "Expected LEN"=w338, "STAT ID"=u8 15, "error in"=w326) -> ("STATs"=w335:T53[], "error out"=w340:errorcluster)  [unwired: 9 in]
                    n87 = call "LEIN CMD read STATs by len.vi"("SID"=w325, "LEIN Variation"=w337, "Expected LEN"=w338, "STAT ID"=u8 5, "error in"=w340) -> ("STATs"=w336:T53[], "error out"=w334:errorcluster)  [unwired: 9 in]
                    n88 = Build Array (concatenate)(w335, w336) -> (w333:T53[])
                    n89 = for {
                      tunnel: [w347] -> w332
                      tunnel: w334 -> [w346]
                      tunnel: w333 -> [w345] mode=indexing
                      tunnel: w330 -> [w342]
                      n90 = call "LEIN Q Uniqe command.vi"("LEIN custom reply Q"=w342, "Retry on err (F)"=TRUE, "Custom Q(F)"=TRUE, "CMD"=w345, "error in"=w346) -> ("error out"=w347:errorcluster)  [unwired: 10 in]
                    }
                  }
                }
              }
              event "Send stroker current pos": Value Change {
                n91 = event-data() -> ("NewVal"=w349:bool)  [unwired: 1 in]
                n92 = case shown="True" w349 {
                  tunnel: [w353 w356] -> w351
                  tunnel: w350 -> [w353 w362]
                  tunnel: "Stroke position to use(mm)" -> [_ w355]
                  frame False {
                  }
                  frame True {
                    w363 = User_Event_List."STROKER tool: Stroker position override sent" ("User Events")
                    n93 = Format Into String(error in=w362, w363) -> (resulting string=w361:string, error out=w364:errorcluster)  [unwired: 2 in]
                    n94 = Number To Fractional String(number=w355) -> (F-format string=w358:string)  [unwired: 3 in]
                    n95 = Concatenate Strings(w361, " position in mm: ", w358) -> (w360:string)
                    n96 = call "Send S&E EVENT message.vi"("Event Source(user)"=S&E_Event_source."User", "Event Description"=w360, "error in (no error)"=w364, "Loc Sub ID/Event ID(No ID)"=w363) -> ("error out"=w357:errorcluster)  [unwired: 10 in, 1 out]
                    n97 = call "Tool Q LEIN stroke fb value ovveride.vi"("stroke value(mm)"=w355, "Serial number(any number(-1))"=i16 -1, "error in (no error)"=w357) -> ("error out"=w356:errorcluster)  [unwired: 12 in]
                  }
                }
              }
              event "Send stroker current pos new": Value Change {
                n98 = event-data() -> ("NewVal"=w367:bool)  [unwired: 1 in]
                n99 = case shown="True" w367 {
                  tunnel: [w371 w378] -> w369
                  tunnel: w368 -> [w371 w384]
                  tunnel: "Stroke pos (mm)" -> [_ w377]
                  frame False {
                  }
                  frame True {
                    w373 = T55 3 items=["Don't change"=3, "On"=1, "Off"=2, "Unknown"=0] ("Stroker enable")
                    w374 = T55 3 items=["Don't change"=3, "On"=1, "Off"=2, "Unknown"=0] ("Stroker direction")
                    w375 = T55 3 items=["Don't change"=3, "On"=1, "Off"=2, "Unknown"=0] ("Anchor")
                    w385 = User_Event_List."STROKER tool: Stroker position override sent" ("User Events")
                    n100 = Format Into String(error in=w384, w385) -> (resulting string=w383:string, error out=w386:errorcluster)  [unwired: 2 in]
                    n101 = Number To Fractional String(number=w377) -> (F-format string=w380:string)  [unwired: 3 in]
                    n102 = Concatenate Strings(w383, " position in mm: ", w380) -> (w382:string)
                    n103 = call "Send S&E EVENT message.vi"("Event Source(user)"=S&E_Event_source."User", "Event Description"=w382, "error in (no error)"=w386, "Loc Sub ID/Event ID(No ID)"=w385) -> ("error out"=w379:errorcluster)  [unwired: 10 in, 1 out]
                    n104 = call "Tool Q LEIN stroke fb value ovveride new.vi"("stroke value(mm)"=w377, "Pos Change"=TRUE, "Serial number(any number(-1))"=i16 -1, "error in (no error)"=w379, "Solenoid 3"=w375, "Solenoid 2"=w374, "Solenoid 1"=w373) -> ("error out"=w378:errorcluster)  [unwired: 8 in]
                  }
                }
              }
              event Value Change {
                w388 = ""
                (unwired) T56 [] ("FW module status codes")
                n105 = event-data() -> ()  [unwired: 1 in, 1 out]
                n106 = local write "Additional Task status"(w388) -> ()
                n107 = local write "Additional Error status"(w388) -> ()
                n108 = local write "Additional Debug status"(w388) -> ()
                "Common error" <- T17 {"Uptime(minutes)"=0, "Com state 1 (crc/Tx)"=0, "Com state 2 (bit timing /Rx)"=0, "System error code"=0, "Module error mask"=0} ("Common error")
                "Common Task status" <- T16 {"Task ID"=0, "Task counter"=0, "Task result code"=0, "reserved"=0} ("Common Task status")
                "Task received" <- FALSE ("Task received")
                "Error received" <- FALSE ("Error received")
                "Debug received" <- FALSE ("Debug received")
                "Common Debug data" <- T18 {"Max handler call interval"=0, "Messages received"=0, "Valid messages received"=0, "Replies sent"=0, "Nack sent"=0} ("Common debug data")
              }
              event "Get Task registers": Value Change {
                n109 = event-data() -> ("NewVal"=w400:bool)  [unwired: 1 in]
                n110 = case shown="True" w400 {
                  tunnel: [w404 w436] -> w402
                  tunnel: w401 -> [w404 w437]
                  tunnel: w399 -> [_ w429]
                  tunnel: w398 -> [_ w424]
                  tunnel: "Node" -> [_ w423]
                  frame False {
                  }
                  frame True {
                    w410 = T16 {"Task ID"=0, "Task counter"=0, "Task result code"=0, "reserved"=0} ("Common Task status")
                    n111 = call <vilib>:"Set Busy.vi"("error in (no error)"=w437) -> ("error out"=w432:errorcluster)  [unwired: 9 in, 1 out]
                    n112 = call "Tool sub node list.vi"("Tool node"=w423, "error in (no error)"=w432) -> ("Main node address"=w405:u8, "Via master"=w426:bool, "LEIN Variation"=w425:T52, "SID"=w427:u8, "Exp len"=w430:T57, "error out"=w431:errorcluster)  [unwired: 6 in, 2 out]
                    n113 = Unbundle By Name(w430) -> ("LEIN 1(Task)"=w428:u16)
                    n114 = call "LEIN CMD read STATs by len.vi"("SID"=w427, "LEIN Variation"=w425, "Expected LEN"=w428, "STAT ID"=u8 1, "error in"=w431) -> ("STATs"=w433:T53[], "error out"=w434:errorcluster)  [unwired: 9 in]
                    n115 = call "Send multipart STAT message and wait for reply.vi"("LEIN custom reply Q"=w429, "Via master"=w426, "Master Address"=w405, "LEIN Variation"=w425, "Multipart message"=w433, "error in"=w434, "timeout per message"=w424) -> ("DATA"=w419:u8[], "Data received"=w417:bool, "error out"=w420:errorcluster)  [unwired: 6 in]
                    n116 = Byte Array To String(unsigned byte array=w419) -> (string=w422:string)
                    n117 = Unflatten From String(type=w410, binary string=w422, byte order (0:big-endian, network order)=T29."little-endian", error in (no error)=w420) -> (rest of the binary string=w412:string, value=w413:T16, error out=w418:errorcluster)  [unwired: 1 in]
                    n118 = call "emi_Is Error.vi"("error in (no error)"=w418) -> ("error out"=w414:errorcluster, "Is Error"=w416:bool)  [unwired: 13 in]
                    n119 = Not(x=w416) -> (.not. x?=w415:bool)
                    n120 = And(x=w415, y=w417) -> (x .and. y?=w411:bool)
                    n121 = case shown="False" w411 {
                      tunnel: w414 -> [w439 w443]
                      tunnel: w413 -> [_ w442]
                      tunnel: w412 -> [_ w441]
                      tunnel: w410 -> [w440 _]
                      tunnel: [w440 w442] -> w409
                      tunnel: [w439 w443] -> w407
                      tunnel: ["" w441] -> w408
                      frame False {
                      }
                      frame True {
                      }
                    }
                    "Additional Task status" <- w408
                    n122 = local write "Task received"(w411) -> ()
                    n123 = local write "Common Task status"(w409) -> ()
                    n124 = call <vilib>:"Clear Errors.vi"("error in (no error)"=w407) -> ("error out"=w406:errorcluster)  [unwired: 6 in]
                    n125 = call <vilib>:"Unset Busy.vi"("error in (no error)"=w406) -> ("error out"=w436:errorcluster)  [unwired: 10 in]
                  }
                }
              }
              event "Get Error registers": Value Change {
                n126 = event-data() -> ("NewVal"=w447:bool)  [unwired: 1 in]
                n127 = local read "Node"() -> (w444:T15)
                n128 = case shown="True" w447 {
                  tunnel: [w451 w483] -> w449
                  tunnel: w448 -> [w451 w484]
                  tunnel: w446 -> [_ w476]
                  tunnel: w445 -> [_ w471]
                  tunnel: w444 -> [_ w470]
                  frame False {
                  }
                  frame True {
                    w456 = T17 {"Uptime(minutes)"=0, "Com state 1 (crc/Tx)"=0, "Com state 2 (bit timing /Rx)"=0, "System error code"=0, "Module error mask"=0} ("Common error")
                    n129 = call <vilib>:"Set Busy.vi"("error in (no error)"=w484) -> ("error out"=w479:errorcluster)  [unwired: 9 in, 1 out]
                    n130 = call "Tool sub node list.vi"("Tool node"=w470, "error in (no error)"=w479) -> ("Main node address"=w452:u8, "Via master"=w473:bool, "LEIN Variation"=w472:T52, "SID"=w474:u8, "Exp len"=w477:T57, "error out"=w478:errorcluster)  [unwired: 6 in, 2 out]
                    n131 = Unbundle By Name(w477) -> ("LEIN 0(error)"=w475:u16)
                    n132 = call "LEIN CMD read STATs by len.vi"("SID"=w474, "LEIN Variation"=w472, "Expected LEN"=w475, "STAT ID"=u8 0, "error in"=w478) -> ("STATs"=w480:T53[], "error out"=w481:errorcluster)  [unwired: 9 in]
                    n133 = call "Send multipart STAT message and wait for reply.vi"("LEIN custom reply Q"=w476, "Via master"=w473, "Master Address"=w452, "LEIN Variation"=w472, "Multipart message"=w480, "error in"=w481, "timeout per message"=w471) -> ("DATA"=w466:u8[], "Data received"=w464:bool, "error out"=w467:errorcluster)  [unwired: 6 in]
                    n134 = Byte Array To String(unsigned byte array=w466) -> (string=w469:string)
                    n135 = Unflatten From String(type=w456, binary string=w469, byte order (0:big-endian, network order)=T29."little-endian", error in (no error)=w467) -> (rest of the binary string=w459:string, value=w460:T17, error out=w465:errorcluster)  [unwired: 1 in]
                    n136 = call "emi_Is Error.vi"("error in (no error)"=w465) -> ("error out"=w461:errorcluster, "Is Error"=w463:bool)  [unwired: 13 in]
                    n137 = Not(x=w463) -> (.not. x?=w462:bool)
                    n138 = And(x=w462, y=w464) -> (x .and. y?=w457:bool)
                    n139 = case shown="True" w457 {
                      tunnel: w461 -> [w486 w490]
                      tunnel: w460 -> [_ w489]
                      tunnel: w459 -> [_ w488]
                      tunnel: w456 -> [w487 _]
                      tunnel: [w487 w489] -> w455
                      tunnel: [w486 w490] -> w454
                      tunnel: ["" w488] -> w458
                      frame False {
                      }
                      frame True {
                      }
                    }
                    "Additional Error status" <- w458
                    n140 = local write "Error received"(w457) -> ()
                    n141 = local write "Common error"(w455) -> ()
                    n142 = call <vilib>:"Clear Errors.vi"("error in (no error)"=w454) -> ("error out"=w453:errorcluster)  [unwired: 6 in]
                    n143 = call <vilib>:"Unset Busy.vi"("error in (no error)"=w453) -> ("error out"=w483:errorcluster)  [unwired: 10 in]
                  }
                }
              }
              event "Clear error": Value Change {
                n144 = event-data() -> ("NewVal"=w494:bool)  [unwired: 1 in]
                n145 = local read "Node"() -> (w491:T15)
                n146 = case shown="True" w494 {
                  tunnel: [w498 w509] -> w496
                  tunnel: w495 -> [w498 w510]
                  tunnel: w493 -> [_ _]
                  tunnel: w492 -> [_ _]
                  tunnel: w491 -> [_ w507]
                  frame False {
                  }
                  frame True {
                    n147 = call <vilib>:"Set Busy.vi"("error in (no error)"=w510) -> ("error out"=w508:errorcluster)  [unwired: 9 in, 1 out]
                    n148 = call "Tool sub node list.vi"("Tool node"=w507, "error in (no error)"=w508) -> ("Main node address"=w499:u8, "Via master"=w501:bool, "LEIN Variation"=w503:T52, "SID"=w502:u8, "error out"=w504:errorcluster)  [unwired: 6 in, 3 out]
                    n149 = call "LEIN CMD send ACTI f2 reset error.vi"("Master"=w499, "Retry on err (F)"=FALSE, "Via master"=w501, "SID"=w502, "LEIN Variation"=w503, "error in (no error)"=w504) -> ("error out"=w505:errorcluster)  [unwired: 9 in]
                    n150 = call <vilib>:"Clear Errors.vi"("error in (no error)"=w505) -> ("error out"=w506:errorcluster)  [unwired: 6 in]
                    n151 = call <vilib>:"Unset Busy.vi"("error in (no error)"=w506) -> ("error out"=w509:errorcluster)  [unwired: 10 in]
                  }
                }
              }
              event "Get Debug registers": Value Change {
                n152 = event-data() -> ("NewVal"=w514:bool)  [unwired: 1 in]
                n153 = local read "Node"() -> (w511:T15)
                n154 = case shown="True" w514 {
                  tunnel: [w518 w550] -> w516
                  tunnel: w515 -> [w518 w551]
                  tunnel: w513 -> [_ w543]
                  tunnel: w512 -> [_ w538]
                  tunnel: w511 -> [_ w537]
                  frame False {
                  }
                  frame True {
                    w523 = T18 {"Max handler call interval"=0, "Messages received"=0, "Valid messages received"=0, "Replies sent"=0, "Nack sent"=0} ("Common debug data")
                    n155 = call <vilib>:"Set Busy.vi"("error in (no error)"=w551) -> ("error out"=w546:errorcluster)  [unwired: 9 in, 1 out]
                    n156 = call "Tool sub node list.vi"("Tool node"=w537, "error in (no error)"=w546) -> ("Main node address"=w519:u8, "Via master"=w540:bool, "LEIN Variation"=w539:T52, "SID"=w541:u8, "Exp len"=w544:T57, "error out"=w545:errorcluster)  [unwired: 6 in, 2 out]
                    n157 = Unbundle By Name(w544) -> ("LEIN 14(Debug)"=w542:u16)
                    n158 = call "LEIN CMD read STATs by len.vi"("SID"=w541, "LEIN Variation"=w539, "Expected LEN"=w542, "STAT ID"=u8 14, "error in"=w545) -> ("STATs"=w547:T53[], "error out"=w548:errorcluster)  [unwired: 9 in]
                    n159 = call "Send multipart STAT message and wait for reply.vi"("LEIN custom reply Q"=w543, "Via master"=w540, "Master Address"=w519, "LEIN Variation"=w539, "Multipart message"=w547, "error in"=w548, "timeout per message"=w538) -> ("DATA"=w533:u8[], "Data received"=w531:bool, "error out"=w534:errorcluster)  [unwired: 6 in]
                    n160 = Byte Array To String(unsigned byte array=w533) -> (string=w536:string)
                    n161 = Unflatten From String(type=w523, binary string=w536, byte order (0:big-endian, network order)=T29."little-endian", error in (no error)=w534) -> (rest of the binary string=w526:string, value=w527:T18, error out=w532:errorcluster)  [unwired: 1 in]
                    n162 = call "emi_Is Error.vi"("error in (no error)"=w532) -> ("error out"=w528:errorcluster, "Is Error"=w530:bool)  [unwired: 13 in]
                    n163 = Not(x=w530) -> (.not. x?=w529:bool)
                    n164 = And(x=w529, y=w531) -> (x .and. y?=w522:bool)
                    n165 = case shown="False" w522 {
                      tunnel: w528 -> [w553 w557]
                      tunnel: w527 -> [_ w556]
                      tunnel: w526 -> [_ w555]
                      tunnel: w523 -> [w554 _]
                      tunnel: [w554 w556] -> w524
                      tunnel: [w553 w557] -> w521
                      tunnel: ["" w555] -> w525
                      frame False {
                      }
                      frame True {
                      }
                    }
                    "Additional Debug status" <- w525
                    n166 = local write "Common Debug data"(w524) -> ()
                    n167 = local write "Debug received"(w522) -> ()
                    n168 = call <vilib>:"Clear Errors.vi"("error in (no error)"=w521) -> ("error out"=w520:errorcluster)  [unwired: 6 in]
                    n169 = call <vilib>:"Unset Busy.vi"("error in (no error)"=w520) -> ("error out"=w550:errorcluster)  [unwired: 10 in]
                  }
                }
              }
              event Timeout {
                n170 = event-data() -> ()  [unwired: 1 in, 2 out]
              }
            }
          }
          frame "Stop" {
            # "Så ikke auto starter igjen om enablet"
            # "To alow VI to exit befor \nAplicatin End.\nFor use in dialogs"
            # "Stop the loop. May be restarted later. Close interfaces and the like"
            n171 = disable-structure shown="Enabled" {
              disable-tunnel: w564 -> [w577 w578]
              disable-tunnel: w563 -> [w576 _]
              disable-tunnel: [w574 w578] -> w562
              frame Enabled {
                n172 = call-poly "emi_SMLoop Control.vi"("Loop ID in"=w576, "Enable"=FALSE, "error in (no error)"=w577) -> ("error out"=w574:errorcluster)  [unwired: 11 in, 1 out]
              }
              frame Disabled {
              }
            }
            n173 = call "emi_FP Hide.vi"("error in (no error)"=w562) -> ("error out"=w561:errorcluster)  [unwired: 13 in, 1 out]
            n174 = disable-structure shown="Disabled" {
              disable-tunnel: w561 -> [w567 w573]
              disable-tunnel: [w566 w573] -> w560
              frame Disabled {
                n175 = call "emi_Get Debug Aditional status.vi"("error in (no error)"=w567) -> ("Debug Additional"=w569:bool, "error out"=w572:errorcluster)  [unwired: 13 in]
                n176 = call "emi_Get Debug Log status.vi"("error in (no error)"=w572) -> ("Debug Log"=w570:bool, "error out"=w571:errorcluster)  [unwired: 13 in]
                n177 = call "emi_Set Debug status.vi"("Debug Disp"=FALSE, "Debug Log"=w570, "Debug Aditional"=w569, "error in (no error)"=w571) -> ("error out"=w566:errorcluster)  [unwired: 11 in]
              }
              frame Enabled {
              }
            }
          }
          frame "Error Handling" {
            # "Loop automaticaly returns here after error is found. If error is cleared, \nLoop wil continue as normal(if was operative when error."
          }
          frame "End" {
            # "Only executes at application end has. Should performa any action the loop \nneeds to finnish. Executes only once."
          }
          frame "Post" {
            # "Only exists to pas true to loop conditional without extra VI. DO Not edit"
          }
        }
      }
      n178 = while {
        shift-right: [w58] -> _
        shift-left: _ -> [w54]
        shift-right: [w56] -> w44
        shift-left: w38 -> [w52]
        tunnel: [w55] -> _
        shift-right: [w53] -> _
        shift-left: _ -> [w48]
        tunnel: w40 -> [w49]
        i -> [w55]
        stop <- w57 stop-if-true
        n179 = call "emi_SMLoop Start.vi"("Loop ID"=w49, "error in (no error)"=w52, "Force Stop(F)"=w48) -> ("Loop command"=w50:T31, "error out"=w51:errorcluster, "Loop ID out"=w47:i32)  [unwired: 10 in]
        n180 = case shown="\"Normal Operation\"" w50 {
          tunnel: [w62 w63 w68 w111 w124 w127 w128 w131] -> w58
          tunnel: [_ _ _ _ _ _ _ TRUE] -> w57
          tunnel: w51 -> [w59 w65 w67 w113 w125 w126 w129 w132]
          tunnel: [w59 w64 w67 w112 w125 w126 w129 w132] -> w56
          tunnel: w54 -> [_ w63 w68 w111 w124 w127 w128 w131]
          tunnel: [w60 _ _ FALSE ("Force End") _ _ _ _] -> w53
          tunnel: w47 -> [_ _ _ _ _ _ _ _]
          frame "Init" {
            w60 = FALSE  # Force end
            w61 = FALSE  # Placeholder
            # "First case that is executed, executes regardless of loop beeing enabled.\nOnly executes once. Init loop data and other variables."
            n181 = Bundle("Placeholder"=w61) -> (w62:cluster{"Placeholder":bool})  [unwired: 1 in]
          }
          frame "Standby", Default {
            # "Case that is executed when the loop is not enabled. Should not be edited."
            n182 = call "emi_Wait MS with err.vi"("milliseconds to wait(0)"=u32 200, "error in (no error)"=w65) -> ("error out"=w64:errorcluster)  [unwired: 13 in]
          }
          frame "Start" {
            # "Start or restart the loop. Should perform any init code. \nOpen channel and so on. Will perform each time the system is restarted."
          }
          frame "Normal Operation" {
            # "Normal Throughput"
            # "All normal tasks belong here. This will be repeated, until error, disable, restart or\nforsed to restart. OBS, reduce overhead with internal loop(will execute unevenly)."
            n183 = call "Get Analog Vars.vi"("Tool"=FALSE, "error in (no error)"=w113) -> ("Analog Vars"=w79:T24[], "error out"=w107:errorcluster)  [unwired: 7 in, 5 out]
            n184 = call "Get Analog Vars.vi"("Tool"=TRUE, "error in (no error)"=w107) -> ("Analog Vars"=w78:T24[], "error out"=w81:errorcluster)  [unwired: 7 in, 5 out]
            n185 = call "Get Modem Status Analog Vars.vi"("error in (no error)"=w81) -> ("Analog Vars"=w77:T24[], "error out"=w80:errorcluster)  [unwired: 8 in, 5 out]
            n186 = call "Get Digital Vars.vi"("Tool"=FALSE, "error in (no error)"=w80) -> ("Analog Vars"=w74:T20[], "error out"=w104:errorcluster)  [unwired: 7 in, 5 out]
            n187 = call "Get Digital Vars.vi"("Tool"=TRUE, "error in (no error)"=w104) -> ("Values"=w82:T58[], "Analog Vars"=w73:T20[], "error out"=w76:errorcluster)  [unwired: 7 in, 4 out]
            n188 = call "Get Modem Status Digital Vars.vi"("error in (no error)"=w76) -> ("Analog Vars"=w72:T20[], "error out"=w75:errorcluster)  [unwired: 8 in, 5 out]
            n189 = call "GS Var Common Ana Fixed Settings.vi"("error in (no error)"=w75) -> ("Common Analog Var Fixed out"=w87:T59[], "Common Digital var Fixed"=w86:T65[], "error out"=w71:errorcluster)  [unwired: 12 in]
            n190 = call "GS Var TOOL Ana Fixed Settings.vi"("error in (no error)"=w71) -> ("Tool Analog var Fixed out"=w88:T59[], "Tool Digital Var Fixed out"=w85:T65[], "error out"=w70:errorcluster)  [unwired: 12 in]
            n191 = call "GS Var Modem Status Ana Fixed Settings.vi"("error in (no error)"=w70) -> ("Modem Status Analog var Fixed out"=w84:T59[], "Modem Status Digital Var Fixed out"=w83:T65[], "error out"=w69:errorcluster)  [unwired: 12 in]
            n192 = Index Array(array=w82, index #1=Variable_List_Tool_Digital."Tool Stroke enable Valve") -> (element #1=→"Solenoid State Master":T58, element #2=→"Solenoid State Stroker":T58, element #3=→"Anchor":T58)  [unwired: 2 in]
            n193 = Build Array (concatenate)(w86, w85, w83) -> (w102:T65[])
            n194 = Build Array (concatenate)(w74, w73, w72) -> (w101:T20[])
            n195 = Build Array (concatenate)(w87, w88, w84) -> (w99:T59[])
            n196 = Build Array (concatenate)(w79, w78, w77) -> (w100:T24[])
            n197 = for {
              tunnel: w99 -> [w118] mode=indexing
              tunnel: w100 -> [w116] mode=indexing
              tunnel: [w115] -> w98 mode=indexing
              n198 = Unbundle By Name(w118) -> ("Name"=w117:string)
              n199 = Bundle By Name(cluster=T23 {"Name"="", "val"={"Value"=nan, "Unit"="", "Status"=0}} ("Cluster"), "Name"=w117, "val"=w116) -> (w115:T23)
            }
            "System analog values" <- w98
            n200 = for {
              tunnel: w102 -> [w123] mode=indexing
              tunnel: w101 -> [w120] mode=indexing
              tunnel: [w119] -> w97 mode=indexing
              n201 = Unbundle By Name(w123) -> ("Name"=w121:string)
              n202 = Bundle By Name(cluster=T19 {"Name"="", "Val"={"ON/OFF TEXT"="OFFLINE", "Val"=1, "Status"=0}} ("Cluster 2"), "Name"=w121, "Val"=w120) -> (w119:T19)
            }
            "System digital values" <- w97
            n203 = call "Tool ID holder.vi"("error in (no error)"=w69) -> ("value out"=→"Main controller":T5, "error out"=w92:errorcluster)  [unwired: 13 in]
            n204 = call "Tool ID holder slaves.vi"("error in (no error)"=w92) -> ("value out"=→"Sub nodes":T5[], "error out"=w93:errorcluster)  [unwired: 13 in]
            n205 = call "emi_Wait until MS multipl with Err.vi"("millisecond multiple(0)"=u32 1000, "error in (no error)"=w93) -> ("error out"=w112:errorcluster)  [unwired: 13 in]
          }
          frame "Stop" {
            # "To alow VI to exit befor \nAplicatin End.\nFor use in dialogs"
            # "Stop the loop. May be restarted later. Close interfaces and the like"
          }
          frame "Error Handling" {
            # "Loop automaticaly returns here after error is found. If error is cleared, \nLoop wil continue as normal(if was operative when error."
          }
          frame "End" {
            # "Only executes at application end has. Should performa any action the loop \nneeds to finnish. Executes only once."
          }
          frame "Post" {
            # "Only exists to pas true to loop conditional without extra VI. DO Not edit"
          }
        }
      }
      n206 = Merge Errors(w45, w44) -> (w43:errorcluster)
    }
  }
  n207 = while "Stat 2 data" {
    shift-right: [w597] -> _
    shift-left: _ -> [w594]
    tunnel: [w595] -> _
    shift-right: [w593] -> _
    shift-left: _ -> [w588]
    tunnel: "LEIN contoller STAT2 data dekoder" -> [w589]
    shift-right: [w586] -> _
    shift-left: "error in (no error)" -> [w592]
    i -> [w595]
    stop <- w596 stop-if-true
    n208 = call "emi_SMLoop Start.vi"("Loop ID"=w589, "error in (no error)"=w592, "Force Stop(F)"=w588) -> ("Loop command"=w590:T31, "error out"=w591:errorcluster, "Loop ID out"=w587:i32)  [unwired: 10 in]
    n209 = case shown="\"Normal Operation\"" w590 {
      tunnel: [w604 w611 w625 w663 w720 w723 w724 w727] -> w597
      tunnel: [_ _ _ _ _ _ _ TRUE] -> w596
      tunnel: w591 -> [w602 w613 w632 w680 w721 w722 w725 w728]
      tunnel: [w601 w612 w618 w678 w721 w722 w725 w728] -> w586
      tunnel: w594 -> [_ w611 w625 w664 w720 w723 w724 w727]
      tunnel: [w610 _ _ FALSE ("Force End") _ _ _ _] -> w593
      tunnel: w587 -> [_ _ _ _ _ _ _ _]
      frame "Init" {
        w598 = u32 0  # Time of last valid tool data
        w606 = 0  # Dig com
        w607 = 0  # Ana com
        w610 = FALSE  # Force end
        # "First case that is executed, executes regardless of loop beeing enabled.\nOnly executes once. Init loop data and other variables."
        n210 = call "Tool LEIN m SIC Controller STAT 2 reply.vi"("error in (no error)"=w602) -> ("notifier out"=w600:refnum<notifier>, "error out"=w601:errorcluster)  [unwired: 13 in]
        n211 = call "emi_Enum Info.vi"("Enum"=Variable_List_Common_Analog."HVPSU Head Voltage" ("Action")) -> ("Numb Elements"=w603:i32)  [unwired: 11 in, 3 out]
        n212 = call "emi_Enum Info.vi"("Enum"=Variable_List_Common_Digital."Tool Connected" ("Action")) -> ("Numb Elements"=w599:i32)  [unwired: 11 in, 3 out]
        n213 = Bundle("notifier out"=w600, "Ana com"=w607, "Dig com"=w606, "Time of last valid tool data"=w598) -> (w605:T69)  [unwired: 1 in]
        n214 = Bundle By Name(cluster=w605, "Ana com"=w603, "Dig com"=w599) -> (w604:T69)
      }
      frame "Standby", Default {
        # "Case that is executed when the loop is not enabled. Should not be edited."
        n215 = call "emi_Wait MS with err.vi"("milliseconds to wait(0)"=u32 50, "error in (no error)"=w613) -> ("error out"=w612:errorcluster)  [unwired: 13 in]
      }
      frame "Start" {
        # "Start or restart the loop. Should perform any init code. Open channel and so on. \nWill perform each time the system is restarted."
        n216 = call "Options GFV.vi"("error in (no error)"=w632) -> ("Options"=w630:T32, "error out"=w631:errorcluster)  [unwired: 16 in, 1 out]
        n217 = Unbundle By Name(w630) -> ("P 7 (Expert).Buffer size"=w628:i32)
        n218 = call "analog Handler.vi"("Action"=Action_Analog_Handler."BUF size(total antal sekund)" ("Action(GET)"), "error in (no error)"=w631, "Start tid / buf size"=w628) -> ("error out"=w624:errorcluster)  [unwired: 7 in, 5 out]
        n219 = call "GS Var TOOL Ana Fixed Settings.vi"("error in (no error)"=w624) -> ("Tool Analog var Fixed out"=w622:T59[], "Tool Digital Var Fixed out"=w621:T65[], "error out"=w623:errorcluster)  [unwired: 12 in]
        n220 = for {
          tunnel: [w644] -> w629
          tunnel: w623 -> [w649]
          tunnel: w622 -> [w648] mode=indexing
          n221 = Unbundle By Name(w648) -> ("ID"=w642:u16, "Maximum upd"=w647:T61)
          n222 = call "analog Handler.vi"("Variable Index"=w642, "Action"=Action_Analog_Handler."REG Variable" ("Action(GET)"), "Upd freq"=w647, "error in (no error)"=w649) -> ("error out"=w645:errorcluster)  [unwired: 6 in, 5 out]
          n223 = call "analog Handler.vi"("Variable Index"=w642, "Action"=Action_Analog_Handler."START Buffer" ("Action(GET)"), "error in (no error)"=w645) -> ("error out"=w644:errorcluster)  [unwired: 7 in, 5 out]
        }
        n224 = call "Status Handler.vi"("Action"=Action_Analog_Handler."BUF size(total antal sekund)", "error in (no error)"=w629, "Start tid(buff size"=w628) -> ("error out"=w626:errorcluster)  [unwired: 8 in, 4 out]
        n225 = for {
          tunnel: [w636] -> w619
          tunnel: w626 -> [w641]
          tunnel: w621 -> [w640] mode=indexing
          n226 = Unbundle By Name(w640) -> ("ID"=w634:u16, "Maximum upd"=w639:T61)
          n227 = call "Status Handler.vi"("Variable Index"=w634, "Action"=Action_Analog_Handler."REG Variable" ("Action(GET)"), "Upd freq"=w639, "error in (no error)"=w641) -> ("error out"=w637:errorcluster)  [unwired: 7 in, 4 out]
          n228 = call "Status Handler.vi"("Variable Index"=w634, "Action"=Action_Analog_Handler."START Buffer" ("Action(GET)"), "error in (no error)"=w637) -> ("error out"=w636:errorcluster)  [unwired: 8 in, 4 out]
        }
        n229 = call "Selected Tool holder.vi"("error in (no error)"=w619) -> ("Tool out"=w616:T50, "error out"=w620:errorcluster)  [unwired: 13 in]
        n230 = To Unsigned Word Integer(number=w616) -> (unsigned 16bit integer=→"Type tab 2":u16)
        n231 = call "Tool information.vi"("Tool in"=w616, "error in (no error)"=w620) -> ("Tool (folder) name"=→"Tool type:":string, "error out"=w618:errorcluster)  [unwired: 10 in, 2 out]
      }
      frame "Normal Operation" {
        w669 = Action_Analog_Handler."SET Value" ("Action(GET)")
        # "v1.14 This case will now set the measurement data to NaN only if the \"Telemetry Timeout Disable\" has\nelapsed."
        # "v1.13 This entire case has been rewritten to allow the Tool connected and the remaning tool variables to have different timeouts\nThe reason why the tool connected variable needs a different timeout than the remaining variables is that the tool connected \nvariable greys out the entire front panel. All other variables are just used for display. \n\nThe tool connected variable has a counter that resets everytime a valid packet from the tool is received. If a valid packet is not received\nduring the last X number of milliseconds, the tool is considered as not connected.\n\nThe remaining variables will be set to NaN on the first received packet timeout"
        # "Tool is connected if data has been received\nfrom the tool in the last X seconds"
        # "This STAT 2 message, comse from the Tool measurement data receiver"
        # "All normal tasks belong here. This will be repeated, until error, disable, restart or\nforsed to restart. OBS, reduce overhead with internal loop(will execute unevenly)."
        n232 = Unbundle By Name(w664) -> ("notifier out"=w677:refnum<notifier>, "Ana com"=w674:i32, "Dig com"=w675:i32)
        n233 = Wait on Notification(notifier=w677, timeout in ms (-1)=2000, error in (no error)=w680) -> (notification=w676:T70, timed out?=w673:bool, error out=w658:errorcluster)  [unwired: 1 in, 1 out]
        n234 = Not(x=w673) -> (.not. x?=w661:bool)
        n235 = call "Predekoder av LEIN stat 2.vi"("Received"=w661, "Cluster"=w676) -> ("Tool analog value"=w660:dbl[], "Tool analog index"=w653:u16[], "Tool digital value"=w659:T58[], "Tool digital indexes"=w652:u16[], "Stroker Raw values"=→"Tool Raw values":T9, "Node status array"=→"Node status array":T6[])  [unwired: 7 in, 1 out]
        n236 = feedback #1() -> (w656:T58[])  [unwired: 1 in]
        n237 = feedback #2() -> (w657:dbl[])  [unwired: 1 in]
        n238 = case shown="False" w661 {
          selector: w661 -> [_ w702]
          tunnel: w664 -> [w698 w705]
          tunnel: [w682 w702] -> w662
          tunnel: [w698 w704] -> w663
          tunnel: w658 -> [w693 w701]
          tunnel: [w692 w701] -> w651
          tunnel: w660 -> [w688 w700]
          tunnel: w659 -> [w685 w699]
          tunnel: [w686 w700] -> w655
          tunnel: [w683 w699] -> w654
          tunnel: w657 -> [w687 _]
          tunnel: w656 -> [w684 _]
          frame False {
            w690 = 1000  # ms
            # "Tool connected timeout"
            n239 = call "Options GFV.vi"("error in (no error)"=w693) -> ("Options"=w695:T32, "error out"=w692:errorcluster)  [unwired: 16 in, 1 out]
            n240 = Unbundle By Name(w698) -> ("Time of last valid tool data"=w696:u32)
            n241 = Unbundle By Name(w695) -> ("P 7 (Expert).Telemetry Timeout Disable"=w691:i32)
            n242 = Tick Count (ms)() -> (millisecond timer value=w697:u32)
            n243 = Multiply(x=w691, y=w690) -> (x*y=w689:i32)
            n244 = Subtract(x=w697, y=w696) -> (x-y=w694:u32)
            n245 = Less?(x=w694, y=w689) -> (x < y?=w682:bool)
            n246 = Not(x=w682) -> (.not. x?=w681:bool)
            n247 = Select(t=w685, s=w681, f=w684) -> (s? t:f=w683:T58[])
            n248 = Select(t=w688, s=w681, f=w687) -> (s? t:f=w686:dbl[])
          }
          frame True {
            # "Valid packet was received.\nReset timer"
            n249 = Tick Count (ms)() -> (millisecond timer value=w703:u32)
            n250 = Bundle By Name(cluster=w705, "Time of last valid tool data"=w703) -> (w704:T69)
          }
        }
        n251 = feedback-in #1(w654) -> ()
        n252 = feedback-in #2(w655) -> ()
        n253 = for {
          tunnel: w651 -> [w712]
          tunnel: [w711] -> w668
          tunnel: w669 -> [w710]
          tunnel: w675 -> [w708]
          tunnel: w654 -> [w707] mode=indexing
          tunnel: w652 -> [w706] mode=indexing
          n254 = Add(x=w708, y=w706) -> (x+y=w709:i32)
          n255 = call "Status Handler.vi"("Variable Index"=w709, "Action"=w710, "Value"=w707, "error in (no error)"=w712) -> ("error out"=w711:errorcluster)  [unwired: 7 in, 4 out]
        }
        n256 = for {
          tunnel: w668 -> [w719]
          tunnel: [w718] -> w650
          tunnel: w669 -> [w717]
          tunnel: w674 -> [w715]
          tunnel: w655 -> [w714] mode=indexing
          tunnel: w653 -> [w713] mode=indexing
          # "Data is sorted when\nwritten to FGV"
          n257 = Add(x=w715, y=w713) -> (x+y=w716:i32)
          n258 = call "analog Handler.vi"("Variable Index"=w716, "Action"=w717, "Value"=w714, "error in (no error)"=w719) -> ("error out"=w718:errorcluster)  [unwired: 6 in, 5 out]
        }
        n259 = call "Bool til status.vi"("Boolean"=w662) -> ("Status"=w667:T58)  [unwired: 8 in]
        n260 = call "Status Handler.vi"("Variable Index"=Variable_List_Common_Digital."Tool Connected" ("Action"), "Action"=Action_Analog_Handler."SET Value", "Value"=w667, "error in (no error)"=w650) -> ("error out"=w678:errorcluster)  [unwired: 7 in, 4 out]
      }
      frame "Stop" {
        # "Stop the loop. May be restarted later. Close interfaces and the like"
      }
      frame "Error Handling" {
        # "Loop automaticaly returns here after error is found. If error is cleared, Loop wil continue\nas normal(if was operative when error."
      }
      frame "End" {
        # "Only executes at application end has. Should performa any action the loop needs to finnish. \nExecutes only once."
      }
      frame "Post" {
        # "Only exists to pas true to loop conditional without extra VI. DO Not edit"
      }
    }
  }
  n261 = call "emi_Dialog End.vi"("error in"=w8) -> ("error out"=w6:errorcluster)  [unwired: 14 in]
  n262 = call <vilib>:"Clear Errors.vi"("error in (no error)"=w6) -> ()  [unwired: 6 in, 1 out]
